vi "LabVIEW Code.vi"() -> ()   [LabVIEW 2017]
uses:
  <vilib>/AWS Toolkit/Core/HTTP Request/AWS Credentials.ctl
  <vilib>/AWS Toolkit/Core/HTTP Request/Region.ctl
  <vilib>/Utility/error.llb/DialogType.ctl
  <vilib>/AWS Toolkit/JSON Parsing/JSON Type.ctl
  <vilib>/DAQmx/read.llb/DAQmx Read (Analog 1D Wfm NChan NSamp).vi
  <extravilib>/ChannelInstances/Tag-bool/Read With Abort.vi
  <extravilib>/ChannelInstances/Tag-bool/Write With Abort.vi
  <extravilib>/ChannelInstances/Tag-bool/Instantiate.vi
  <vilib>/VirtualBench/_PS Configure Voltage Output2.vi
  <vilib>/VirtualBench/_PS Configure Voltage Output1.vi
  <vilib>/VirtualBench/_DMM Configure Measurement6.vi
  <vilib>/VirtualBench/_FGEN Configure Standard Waveform30.vi
  <vilib>/Waveform/WDTFileIO.llb/Export Waveforms To Spreadsheet File (1D).vi
  <vilib>/DAQmx/create/channels.llb/DAQmx Create Channel (AI-Voltage-Basic).vi
  <vilib>/DAQmx/configure/timing.llb/DAQmx Timing (Sample Clock).vi
  <vilib>/DAQmx/miscellaneous.llb/DAQmx Fill In Error Info.vi
  <extravilib>/ChannelInstances/Tag-bool/EndpointRead.vi
  <extravilib>/ChannelInstances/Tag-bool/Endpoint.vi
  <vilib>/AWS Toolkit/IoT/IoT Session/IoT Session.lvclass
  <vilib>/AWS Toolkit/Core/HTTP Request/HTTP Request.lvclass
  <vilib>/AWS Toolkit/IoT/Thing Shadow/Thing Shadow.lvclass
  <vilib>/AWS Toolkit/JSON Parsing/NI_JSON Parsing.lvlib
  <vilib>/VirtualBench/VirtualBench.lvlib
  <extravilib>/ChannelInstances/Tag-bool.lvlib
panel:
  in  "Physical Channel":tag="Dev1/ai0"
  out "usbAcquire":string
  out "Reset":string
  out "msoAcquire":string
  out "VB Name":string="False"
  out "FGen Waveform":string="False"
  out "FGen Waveform":i32
  out "DMM Measurement":dbl caption="Measurement"
  out "DIOUpdateValue":string
  out "DIOPins":tag
  out "pin 7":string
  out "pin 6":string
  out "pin 5":string
  out "pin 4":string
  out "pin 3":string
  out "pin 2":string
  out "pin 1":string
  out "pin 0":string
  out "stopProgramme":string
  out "Alexa Stop":bool=TRUE
  out "DMM Range":dbl caption="Range"
  out "Needs Updating":bool=TRUE
  out "Device Name":tag="VB8012-308BD6C"
  out "Current Update Value":dbl
  out "Update":i32
  out "Voltage Update Value":dbl
  out "Voltage Channel":tag="ps/+6V"
  in  "Auto Range":bool=TRUE
  out "DMM Function String":string
  in  "DMM Function":i32
  out "Current C1":dbl
  out "Current C3":dbl
  out "Current C2":dbl
  out "Voltage C3":dbl
  out "Voltage C2":dbl
  out "Voltage C1":dbl
  out "output string":string
  in  "stop":bool
  out "Raw JSON":string
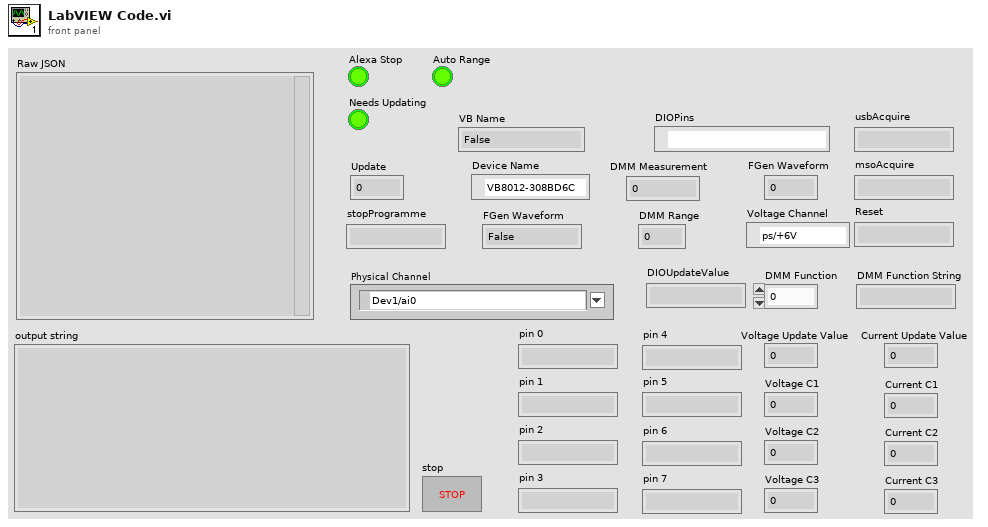
[diagram p1: front panel]
types:
  T1 = typedef "NI_AWS_Core.lvlib/HTTP Request.lvclass/Region.ctl" = enum16{"us-east-1", "us-east-2", "us-west-1", "us-west-2", "ap-northeast-1", "ap-northeast-2", "ap-southeast-1", "ap-southeast-2", "ca-central-1", "eu-central-1", "eu-west-1", "eu-west-2", "sa-east-1"}
  T2 = typedef "NI_AWS_Core.lvlib/HTTP Request.lvclass/AWS Credentials.ctl" = cluster{"Access Key":string, "Secret Key":string}
  T3 = typedef "NI_JSON Parsing.lvlib/JSON Type.ctl" = enum16{"String", "Numeric", "Boolean"}
  T4 = typedef "NI_JSON Parsing.lvlib/Name-Value with Type.ctl" = cluster{"Name Value Pair":T5, "JSON Type":T3}
  T5 = typedef "NI_JSON Parsing.lvlib/Name Value Pair.ctl" = cluster{"name":string, "value":string}
  T6 = cluster{cluster{string, "NumText.Text":string}, "JSON Type":T3}
  T7 = cluster{cluster{string, "NumText.Text":string}, "JSON Type":T3}[]
  T8 = cluster{cluster{string, "DMM Function String":string}, "JSON Type":T3}
  T9 = cluster{cluster{string, "DMM Function String":string}, "JSON Type":T3}[]
  T10 = cluster{cluster{string, string}, "JSON Type":T3}[]
  T11 = cluster{cluster{string, "pin 0":string}, "JSON Type":T3}
  T12 = cluster{cluster{string, "pin 0":string}, "JSON Type":T3}[]
  T13 = cluster{cluster{string, "pin 1":string}, "JSON Type":T3}
  T14 = cluster{cluster{string, "pin 1":string}, "JSON Type":T3}[]
  T15 = cluster{cluster{string, "pin 2":string}, "JSON Type":T3}
  T16 = cluster{cluster{string, "pin 2":string}, "JSON Type":T3}[]
  T17 = cluster{cluster{string, "pin 3":string}, "JSON Type":T3}
  T18 = cluster{cluster{string, "pin 3":string}, "JSON Type":T3}[]
  T19 = cluster{cluster{string, "pin 4":string}, "JSON Type":T3}
  T20 = cluster{cluster{string, "pin 4":string}, "JSON Type":T3}[]
  T21 = cluster{cluster{string, "pin 5":string}, "JSON Type":T3}
  T22 = cluster{cluster{string, "pin 5":string}, "JSON Type":T3}[]
  T23 = cluster{cluster{string, "pin 6":string}, "JSON Type":T3}
  T24 = cluster{cluster{string, "pin 6":string}, "JSON Type":T3}[]
  T25 = cluster{cluster{string, "pin 7":string}, "JSON Type":T3}
  T26 = cluster{cluster{string, "pin 7":string}, "JSON Type":T3}[]
  T27 = cluster{cluster{string, "msoAcquire":string}, "JSON Type":T3}
  T28 = cluster{cluster{string, "msoAcquire":string}, "JSON Type":T3}[]
  T29 = cluster{cluster{string, "usbAcquire":string}, "JSON Type":T3}
  T30 = cluster{cluster{string, "usbAcquire":string}, "JSON Type":T3}[]
  T31 = cluster{cluster{string, "Reset":string}, "JSON Type":T3}
  T32 = cluster{cluster{string, "Reset":string}, "JSON Type":T3}[]
  T33 = cluster{"output string":string, "output string":string}
  T34 = cluster{cluster{"output string":string, "output string":string}, "JSON Type":T3}
  T35 = cluster{cluster{"output string":string, "output string":string}, "JSON Type":T3}[]
  T36 = typedef "Tag-bool.lvlib/))Channel.ctl" = refnum<queue>
  T37 = typedef "DialogType.ctl" = u16
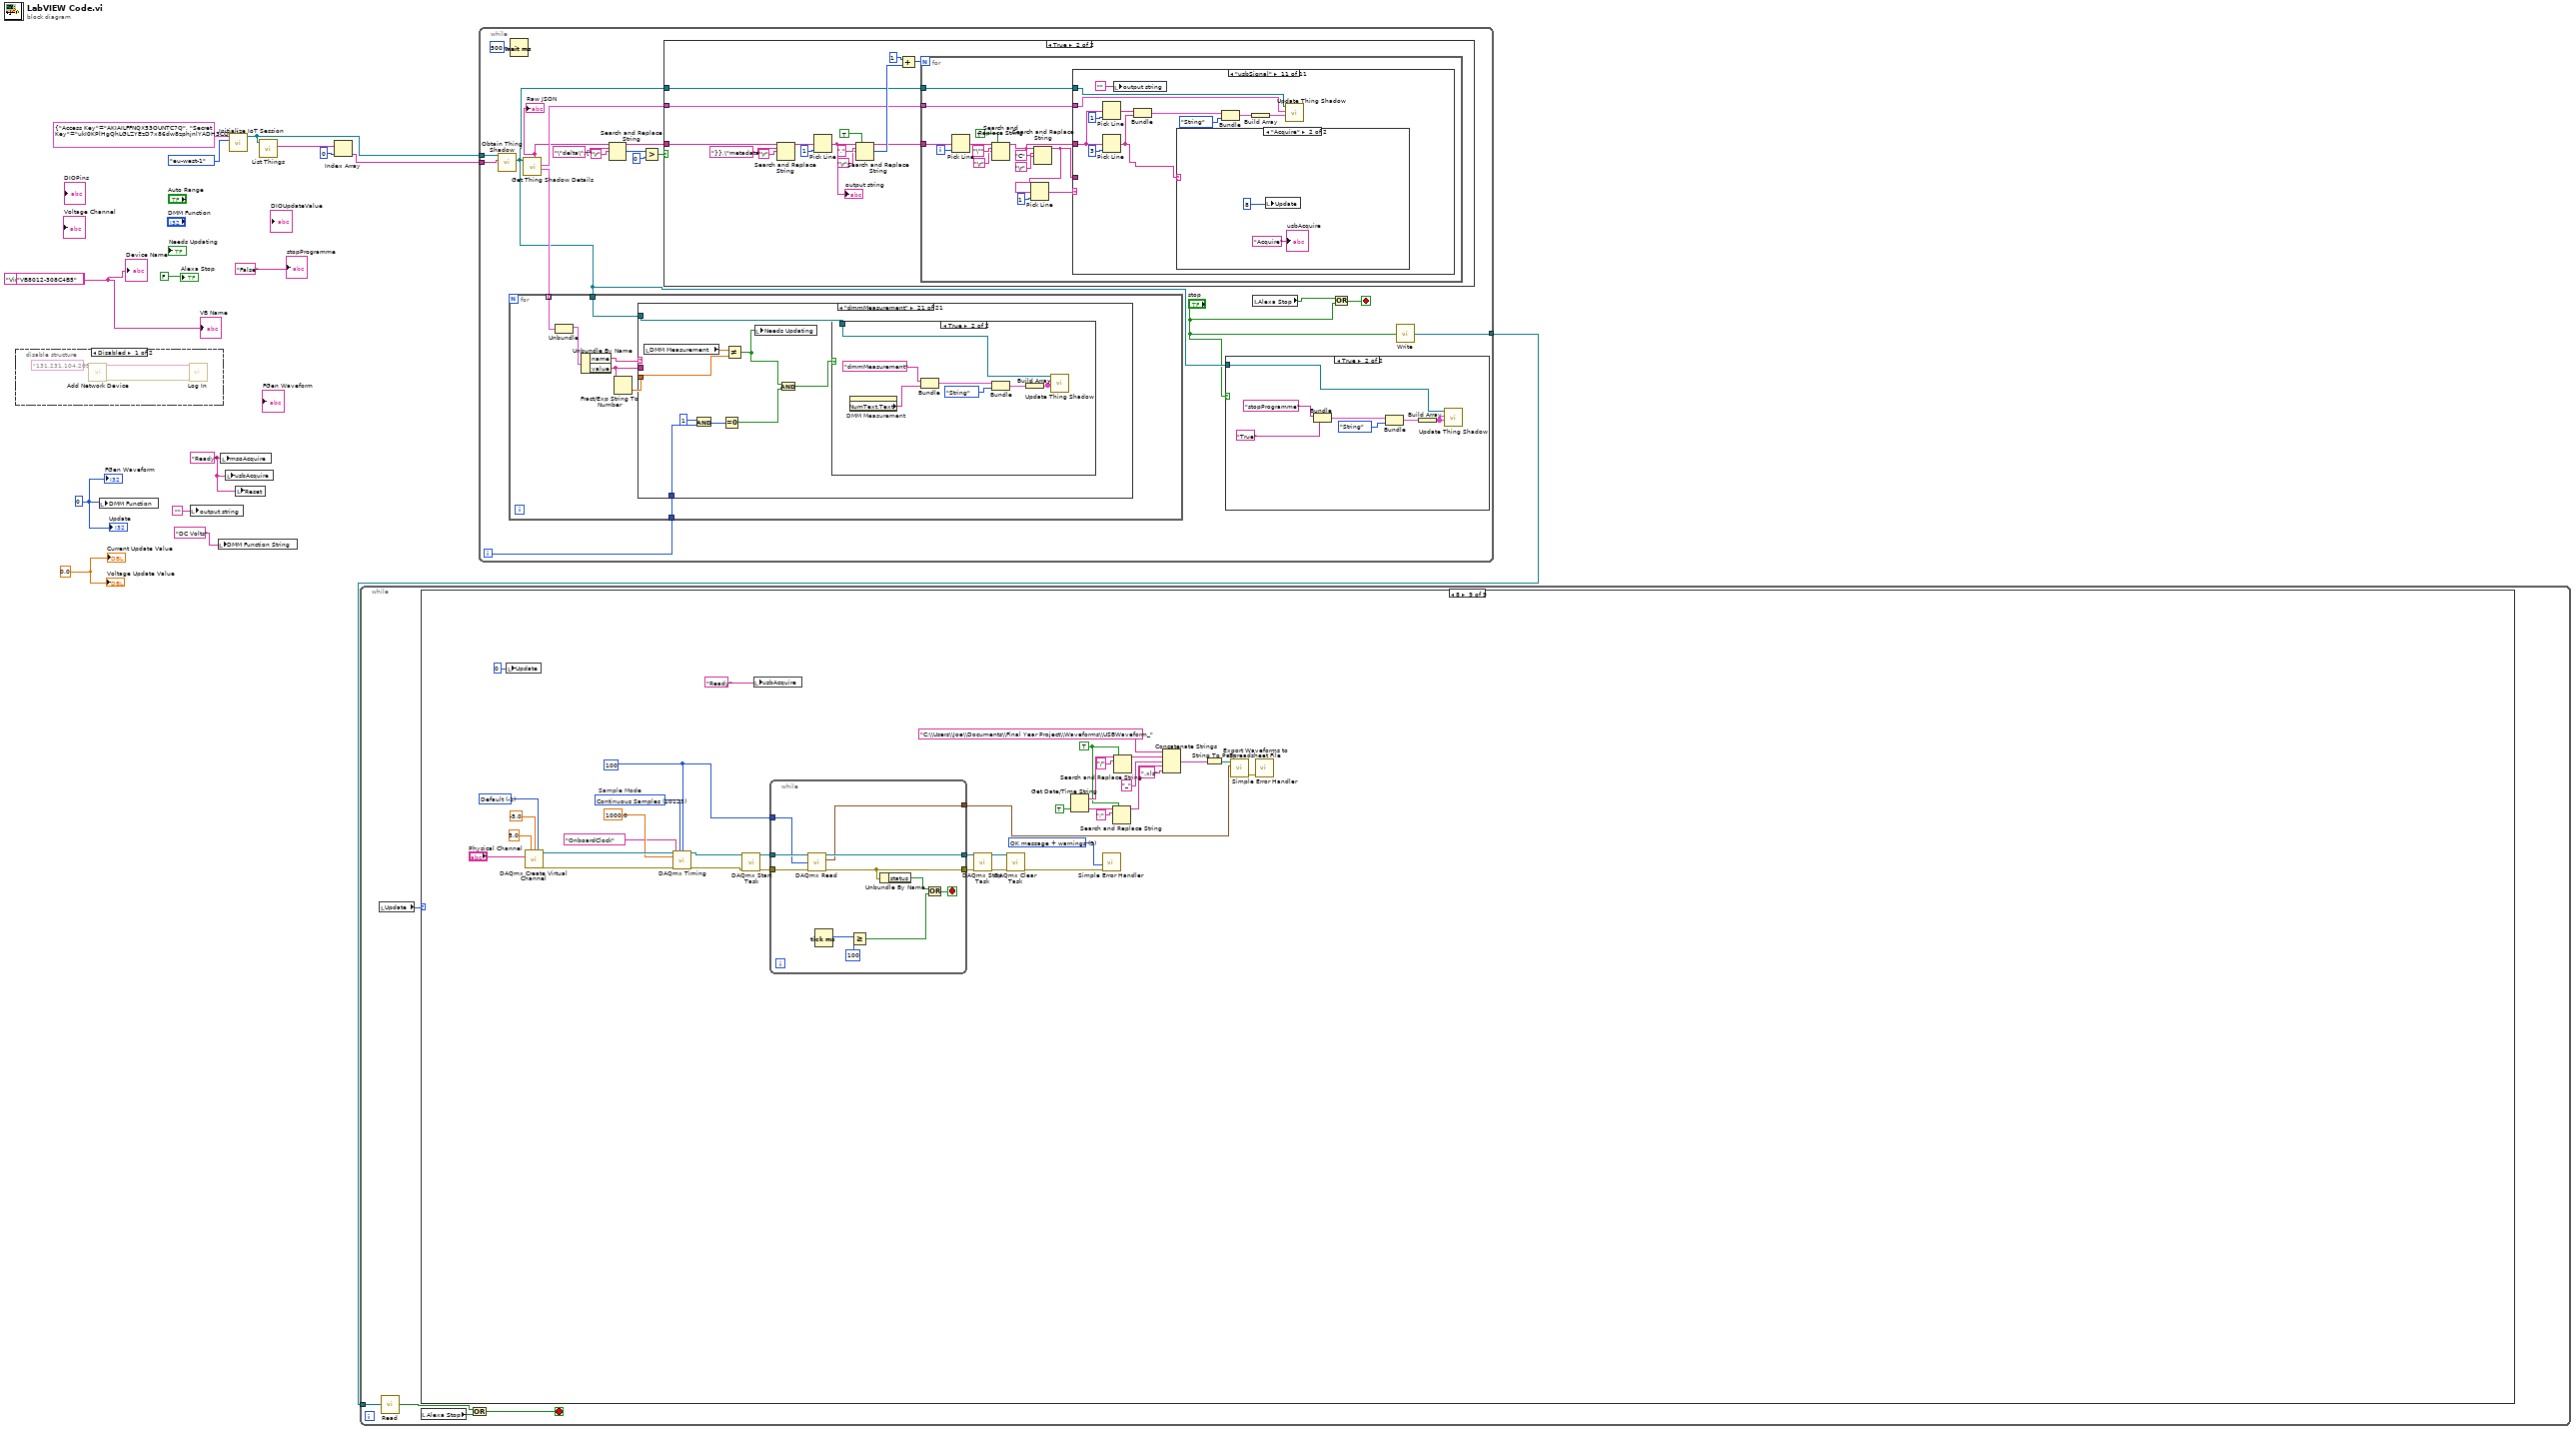
[diagram p0: block diagram]
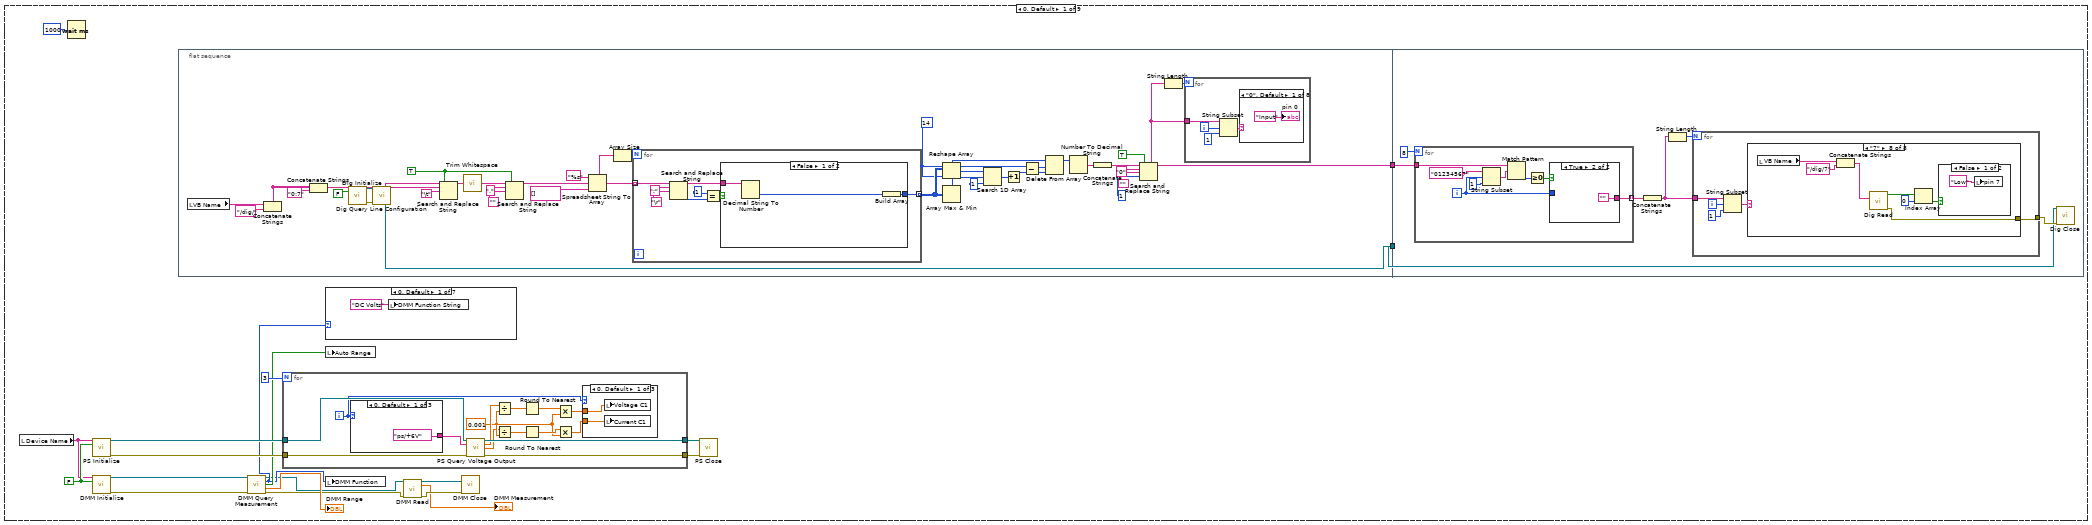
[diagram p3: hidden frame]
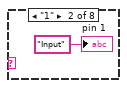
[diagram p4: hidden frame]
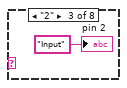
[diagram p5: hidden frame]
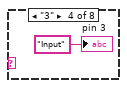
[diagram p6: hidden frame]
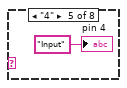
[diagram p7: hidden frame]
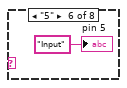
[diagram p8: hidden frame]
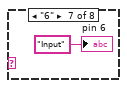
[diagram p9: hidden frame]
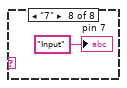
[diagram p10: hidden frame]
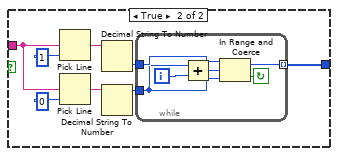
[diagram p11: hidden frame]
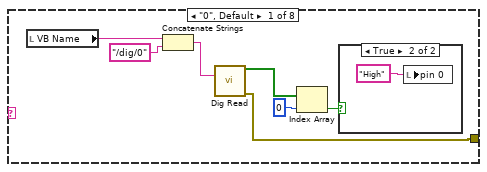
[diagram p12: hidden frame]
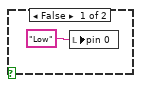
[diagram p13: hidden frame]
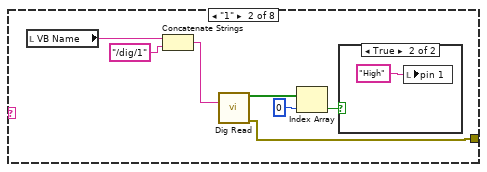
[diagram p14: hidden frame]
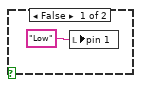
[diagram p15: hidden frame]
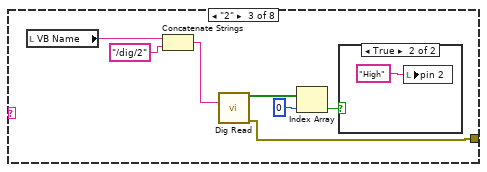
[diagram p16: hidden frame]
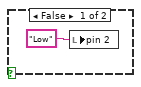
[diagram p17: hidden frame]
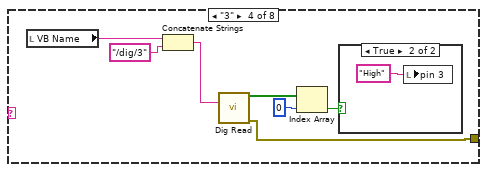
[diagram p18: hidden frame]
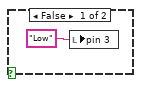
[diagram p19: hidden frame]
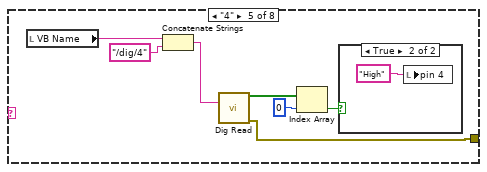
[diagram p20: hidden frame]
diagram:
  w1 = "Ready"
  w2 = tag "VirtualBench-Tank-1" ("Device Name")
  (unwired) tag "VB8012-308C4B5" ("Device Name")
  w8 = 0
  w7 = 0.0
  n1 = disable-structure shown="Disabled" {
    frame Disabled {
      n2 = call <vilib>:"Add Network Device.vi"("IP Or Hostname"="131.231.104.203") -> ("Device"=w18:tag, "Error Out"=w16:errorcluster)  [unwired: 13 in]
      n3 = call <vilib>:"Log In.vi"("Device"=w18, "Error In"=w16) -> ()  [unwired: 13 in, 1 out]
    }
    frame Enabled {
    }
  }
  n4 = local write "DMM Function"(w8) -> ()
  n5 = local write "output string"("") -> ()
  n6 = local write "DMM Function String"("DC Volts") -> ()
  n7 = local write "msoAcquire"(w1) -> ()
  n8 = local write "usbAcquire"(w1) -> ()
  n9 = call <vilib>:"Initialize IoT Session.vi"("Region"=Region."eu-west-1", "AWS Credentials"=T2 {"Access Key"="AKIAILFFNQX53OUNTC7Q", "Secret Key"="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"}) -> ("IoT Session"=w10:refnum<class "IoT Session.lvclass">)  [unwired: 8 in, 1 out]
  n10 = local write "Reset"(w1) -> ()
  n11 = call <vilib>:"List Things.vi"("IoT Session in"=w10) -> ("Things"=w13:string[])  [unwired: 8 in, 2 out]
  n12 = Index Array(array=w13, index=0) -> (element=w11:string)
  n13 = while {
    tunnel: w10 -> [w36]
    tunnel: w11 -> [w35]
    tunnel: [w20] -> w3
    i -> [w19]
    stop <- w24 stop-if-true
    n14 = call <vilib>:"Obtain Thing Shadow.vi"("Thing Name"=w35, "IoT Session in"=w36) -> ("Shadow Thing"=w22:refnum<class "Thing Shadow.lvclass">)  [unwired: 7 in, 2 out]
    n15 = Wait (ms)(milliseconds to wait=u32 500) -> ()  [unwired: 1 out]
    n16 = call <vilib>:"Get Thing Shadow Details.vi"("Thing Shadow in"=w22) -> ("Reported State"=w26:T4[], "Desired State"=w27:T4[], "Raw JSON"=w25:string)  [unwired: 5 in, 3 out]
    "Raw JSON" <- w25
    n17 = for {
      tunnel: w26 -> [w50] mode=indexing
      tunnel: w22 -> [w46]
      tunnel: w19 -> [w44]
      n18 = Unbundle(w50) -> ("Name Value Pair"=w49:T5)  [unwired: 1 out]
      n19 = Unbundle By Name(w49) -> ("name"=w48:string, "value"=w45:string)
      n20 = Fract/Exp String To Number(string=w45) -> (number=w47:dbl)  [unwired: 3 in, 1 out]
      n21 = case shown="\"dmmMeasurement\"" w48 {
        tunnel: w47 -> [_ w53 w64 w75 w86 w97 w108 _ _ _ _ _ _ _ _ _ _ _ _ _ w315]
        tunnel: w46 -> [_ w51 w62 w73 w84 w95 w106 w118 w133 w148 w163 w178 w193 w208 w223 w238 w253 w268 w283 w298 w314]
        tunnel: w45 -> [_ _ _ _ _ _ _ w117 w132 w147 w162 w177 w192 w207 w222 w237 w252 w267 w282 w297 _]
        tunnel: w44 -> [_ _ _ _ _ _ _ _ _ _ _ _ _ _ _ _ _ _ _ _ w313]
        frame "j", Default {
        }
        frame "voltageC1" {
          n22 = local read "Voltage C1"() -> (w54:dbl)
          n23 = Not Equal?(x=w54, y=w53) -> (x != y?=w52:bool)
          n24 = local write "Needs Updating"(w52) -> ()
          n25 = case shown="True" w52 {
            tunnel: w51 -> [_ w57]
            frame False {
            }
            frame True {
              n26 = property on="Voltage C1" class="DigNum (strict)"() -> ("NumText.Text"=w56:string)  [unwired: 2 in, 2 out]
              n27 = Bundle("voltageC1", "NumText.Text"=w56) -> (w59:cluster{string, "NumText.Text":string})  [unwired: 1 in]
              n28 = Bundle(w59, "JSON Type"=JSON_Type."String") -> (w58:T6)  [unwired: 1 in]
              n29 = Build Array(w58) -> (w61:T7)
              n30 = call <vilib>:"Update Thing Shadow.vi"("Reported State"=w61, "Desired State"=w61, "Thing Shadow in"=w57) -> ()  [unwired: 7 in, 2 out]
            }
          }
        }
        frame "voltageC2" {
          n31 = local read "Voltage C2"() -> (w65:dbl)
          n32 = Not Equal?(x=w65, y=w64) -> (x != y?=w63:bool)
          n33 = local write "Needs Updating"(w63) -> ()
          n34 = case shown="False" w63 {
            tunnel: w62 -> [_ w68]
            frame False {
            }
            frame True {
              n35 = property on="Voltage C2" class="DigNum (strict)"() -> ("NumText.Text"=w67:string)  [unwired: 2 in, 2 out]
              n36 = Bundle("voltageC2", "NumText.Text"=w67) -> (w70:cluster{string, "NumText.Text":string})  [unwired: 1 in]
              n37 = Bundle(w70, "JSON Type"=JSON_Type."String") -> (w69:T6)  [unwired: 1 in]
              n38 = Build Array(w69) -> (w72:T7)
              n39 = call <vilib>:"Update Thing Shadow.vi"("Reported State"=w72, "Desired State"=w72, "Thing Shadow in"=w68) -> ()  [unwired: 7 in, 2 out]
            }
          }
        }
        frame "voltageC3" {
          n40 = local read "Voltage C3"() -> (w76:dbl)
          n41 = Not Equal?(x=w76, y=w75) -> (x != y?=w74:bool)
          n42 = local write "Needs Updating"(w74) -> ()
          n43 = case shown="True" w74 {
            tunnel: w73 -> [_ w79]
            frame False {
            }
            frame True {
              n44 = property on="Voltage C3" class="DigNum (strict)"() -> ("NumText.Text"=w78:string)  [unwired: 2 in, 2 out]
              n45 = Bundle("voltageC3", "NumText.Text"=w78) -> (w81:cluster{string, "NumText.Text":string})  [unwired: 1 in]
              n46 = Bundle(w81, "JSON Type"=JSON_Type."String") -> (w80:T6)  [unwired: 1 in]
              n47 = Build Array(w80) -> (w83:T7)
              n48 = call <vilib>:"Update Thing Shadow.vi"("Reported State"=w83, "Desired State"=w83, "Thing Shadow in"=w79) -> ()  [unwired: 7 in, 2 out]
            }
          }
        }
        frame "currentC1" {
          n49 = local read "Current C1"() -> (w87:dbl)
          n50 = Not Equal?(x=w87, y=w86) -> (x != y?=w85:bool)
          n51 = local write "Needs Updating"(w85) -> ()
          n52 = case shown="True" w85 {
            tunnel: w84 -> [_ w90]
            frame False {
            }
            frame True {
              n53 = property on="Current C1" class="DigNum (strict)"() -> ("NumText.Text"=w89:string)  [unwired: 2 in, 2 out]
              n54 = Bundle("currentC1", "NumText.Text"=w89) -> (w92:cluster{string, "NumText.Text":string})  [unwired: 1 in]
              n55 = Bundle(w92, "JSON Type"=JSON_Type."String") -> (w91:T6)  [unwired: 1 in]
              n56 = Build Array(w91) -> (w94:T7)
              n57 = call <vilib>:"Update Thing Shadow.vi"("Reported State"=w94, "Desired State"=w94, "Thing Shadow in"=w90) -> ()  [unwired: 7 in, 2 out]
            }
          }
        }
        frame "currentC2" {
          n58 = local read "Current C2"() -> (w98:dbl)
          n59 = Not Equal?(x=w98, y=w97) -> (x != y?=w96:bool)
          n60 = local write "Needs Updating"(w96) -> ()
          n61 = case shown="True" w96 {
            tunnel: w95 -> [_ w101]
            frame False {
            }
            frame True {
              n62 = property on="Current C2" class="DigNum (strict)"() -> ("NumText.Text"=w100:string)  [unwired: 2 in, 2 out]
              n63 = Bundle("currentC2", "NumText.Text"=w100) -> (w103:cluster{string, "NumText.Text":string})  [unwired: 1 in]
              n64 = Bundle(w103, "JSON Type"=JSON_Type."String") -> (w102:T6)  [unwired: 1 in]
              n65 = Build Array(w102) -> (w105:T7)
              n66 = call <vilib>:"Update Thing Shadow.vi"("Reported State"=w105, "Desired State"=w105, "Thing Shadow in"=w101) -> ()  [unwired: 7 in, 2 out]
            }
          }
        }
        frame "currentC3" {
          n67 = local read "Current C3"() -> (w109:dbl)
          n68 = Not Equal?(x=w109, y=w108) -> (x != y?=w107:bool)
          n69 = local write "Needs Updating"(w107) -> ()
          n70 = case shown="True" w107 {
            tunnel: w106 -> [_ w110]
            frame False {
            }
            frame True {
              n71 = property on="Current C3" class="DigNum (strict)"() -> ("NumText.Text"=w112:string)  [unwired: 2 in, 2 out]
              n72 = Bundle("currentC3", "NumText.Text"=w112) -> (w114:cluster{string, "NumText.Text":string})  [unwired: 1 in]
              n73 = Bundle(w114, "JSON Type"=JSON_Type."String") -> (w113:T6)  [unwired: 1 in]
              n74 = Build Array(w113) -> (w116:T7)
              n75 = call <vilib>:"Update Thing Shadow.vi"("Reported State"=w116, "Desired State"=w116, "Thing Shadow in"=w110) -> ()  [unwired: 7 in, 2 out]
            }
          }
        }
        frame "dmmFunction" {
          n76 = local read "DMM Function String"() -> (w120:string)
          n77 = Not Equal?(x=w120, y=w117) -> (x != y?=w119:bool)
          n78 = local write "Needs Updating"(w119) -> ()
          n79 = case shown="True" w119 {
            tunnel: w118 -> [_ w123]
            frame False {
            }
            frame True {
              n80 = local read "DMM Function String"() -> (w122:string)
              n81 = Bundle("dmmFunction", "DMM Function String"=w122) -> (w126:cluster{string, "DMM Function String":string})  [unwired: 1 in]
              n82 = Bundle(w126, "JSON Type"=JSON_Type."String") -> (w125:T8)  [unwired: 1 in]
              n83 = Build Array(w125) -> (w121:T9)
              n84 = call <vilib>:"Update Thing Shadow.vi"("Reported State"=w121, "Desired State"=w121, "Thing Shadow in"=w123) -> ()  [unwired: 7 in, 2 out]
            }
          }
        }
        frame "stopProgramme" {
          n85 = local read "stopProgramme"() -> (w134:string)
          n86 = local read "Alexa Stop"() -> (w129:bool)
          n87 = Not Equal?(x=w134, y=w132) -> (x != y?=w131:bool)
          n88 = Not(x=w129) -> (.not. x?=w128:bool)
          n89 = local write "Needs Updating"(w131) -> ()
          n90 = And(x=w131, y=w128) -> (x .and. y?=w130:bool)
          n91 = case shown="True" w130 {
            tunnel: w133 -> [_ w138]
            frame False {
            }
            frame True {
              n92 = local write "output string"("") -> ()
              n93 = Bundle("stopProgramme", "False") -> (w141:cluster{string, string})  [unwired: 1 in]
              n94 = Bundle(w141, "JSON Type"=JSON_Type."String") -> (w140:cluster{cluster{string, string}, "JSON Type":T3})  [unwired: 1 in]
              n95 = Build Array(w140) -> (w137:T10)
              n96 = call <vilib>:"Update Thing Shadow.vi"("Reported State"=w137, "Desired State"=w137, "Thing Shadow in"=w138) -> ()  [unwired: 7 in, 2 out]
            }
          }
        }
        frame "pinC0" {
          n97 = local read "Alexa Stop"() -> (w144:bool)
          n98 = local read "pin 0"() -> (w149:string)
          n99 = Not Equal?(x=w149, y=w147) -> (x != y?=w146:bool)
          n100 = Not(x=w144) -> (.not. x?=w143:bool)
          n101 = local write "Needs Updating"(w146) -> ()
          n102 = And(x=w146, y=w143) -> (x .and. y?=w145:bool)
          n103 = case shown="True" w145 {
            tunnel: w148 -> [_ w157]
            frame False {
            }
            frame True {
              n104 = local read "pin 0"() -> (w150:string)
              n105 = local write "output string"("") -> ()
              n106 = Bundle("pinC0", "pin 0"=w150) -> (w155:cluster{string, "pin 0":string})  [unwired: 1 in]
              n107 = Bundle(w155, "JSON Type"=JSON_Type."String") -> (w154:T11)  [unwired: 1 in]
              n108 = Build Array(w154) -> (w152:T12)
              n109 = call <vilib>:"Update Thing Shadow.vi"("Reported State"=w152, "Desired State"=w152, "Thing Shadow in"=w157) -> ()  [unwired: 7 in, 2 out]
            }
          }
        }
        frame "pinC1" {
          n110 = local read "Alexa Stop"() -> (w159:bool)
          n111 = local read "pin 1"() -> (w164:string)
          n112 = Not Equal?(x=w164, y=w162) -> (x != y?=w161:bool)
          n113 = Not(x=w159) -> (.not. x?=w158:bool)
          n114 = local write "Needs Updating"(w161) -> ()
          n115 = And(x=w161, y=w158) -> (x .and. y?=w160:bool)
          n116 = case shown="True" w160 {
            tunnel: w163 -> [_ w168]
            frame False {
            }
            frame True {
              n117 = local read "pin 1"() -> (w165:string)
              n118 = local write "output string"("") -> ()
              n119 = Bundle("pinC1", "pin 1"=w165) -> (w171:cluster{string, "pin 1":string})  [unwired: 1 in]
              n120 = Bundle(w171, "JSON Type"=JSON_Type."String") -> (w170:T13)  [unwired: 1 in]
              n121 = Build Array(w170) -> (w167:T14)
              n122 = call <vilib>:"Update Thing Shadow.vi"("Reported State"=w167, "Desired State"=w167, "Thing Shadow in"=w168) -> ()  [unwired: 7 in, 2 out]
            }
          }
        }
        frame "pinC2" {
          n123 = local read "Alexa Stop"() -> (w174:bool)
          n124 = local read "pin 2"() -> (w179:string)
          n125 = Not Equal?(x=w179, y=w177) -> (x != y?=w176:bool)
          n126 = Not(x=w174) -> (.not. x?=w173:bool)
          n127 = local write "Needs Updating"(w176) -> ()
          n128 = And(x=w176, y=w173) -> (x .and. y?=w175:bool)
          n129 = case shown="True" w175 {
            tunnel: w178 -> [_ w183]
            frame False {
            }
            frame True {
              n130 = local read "pin 2"() -> (w180:string)
              n131 = local write "output string"("") -> ()
              n132 = Bundle("pinC2", "pin 2"=w180) -> (w186:cluster{string, "pin 2":string})  [unwired: 1 in]
              n133 = Bundle(w186, "JSON Type"=JSON_Type."String") -> (w185:T15)  [unwired: 1 in]
              n134 = Build Array(w185) -> (w182:T16)
              n135 = call <vilib>:"Update Thing Shadow.vi"("Reported State"=w182, "Desired State"=w182, "Thing Shadow in"=w183) -> ()  [unwired: 7 in, 2 out]
            }
          }
        }
        frame "pinC3" {
          n136 = local read "Alexa Stop"() -> (w189:bool)
          n137 = local read "pin 3"() -> (w194:string)
          n138 = Not Equal?(x=w194, y=w192) -> (x != y?=w191:bool)
          n139 = Not(x=w189) -> (.not. x?=w188:bool)
          n140 = local write "Needs Updating"(w191) -> ()
          n141 = And(x=w191, y=w188) -> (x .and. y?=w190:bool)
          n142 = case shown="True" w190 {
            tunnel: w193 -> [_ w198]
            frame False {
            }
            frame True {
              n143 = local read "pin 3"() -> (w195:string)
              n144 = local write "output string"("") -> ()
              n145 = Bundle("pinC3", "pin 3"=w195) -> (w201:cluster{string, "pin 3":string})  [unwired: 1 in]
              n146 = Bundle(w201, "JSON Type"=JSON_Type."String") -> (w200:T17)  [unwired: 1 in]
              n147 = Build Array(w200) -> (w197:T18)
              n148 = call <vilib>:"Update Thing Shadow.vi"("Reported State"=w197, "Desired State"=w197, "Thing Shadow in"=w198) -> ()  [unwired: 7 in, 2 out]
            }
          }
        }
        frame "pinC4" {
          n149 = local read "Alexa Stop"() -> (w204:bool)
          n150 = local read "pin 4"() -> (w209:string)
          n151 = Not Equal?(x=w209, y=w207) -> (x != y?=w206:bool)
          n152 = Not(x=w204) -> (.not. x?=w203:bool)
          n153 = local write "Needs Updating"(w206) -> ()
          n154 = And(x=w206, y=w203) -> (x .and. y?=w205:bool)
          n155 = case shown="True" w205 {
            tunnel: w208 -> [_ w213]
            frame False {
            }
            frame True {
              n156 = local read "pin 4"() -> (w210:string)
              n157 = local write "output string"("") -> ()
              n158 = Bundle("pinC4", "pin 4"=w210) -> (w216:cluster{string, "pin 4":string})  [unwired: 1 in]
              n159 = Bundle(w216, "JSON Type"=JSON_Type."String") -> (w215:T19)  [unwired: 1 in]
              n160 = Build Array(w215) -> (w212:T20)
              n161 = call <vilib>:"Update Thing Shadow.vi"("Reported State"=w212, "Desired State"=w212, "Thing Shadow in"=w213) -> ()  [unwired: 7 in, 2 out]
            }
          }
        }
        frame "pinC5" {
          n162 = local read "Alexa Stop"() -> (w219:bool)
          n163 = local read "pin 5"() -> (w224:string)
          n164 = Not Equal?(x=w224, y=w222) -> (x != y?=w221:bool)
          n165 = Not(x=w219) -> (.not. x?=w218:bool)
          n166 = local write "Needs Updating"(w221) -> ()
          n167 = And(x=w221, y=w218) -> (x .and. y?=w220:bool)
          n168 = case shown="True" w220 {
            tunnel: w223 -> [_ w228]
            frame False {
            }
            frame True {
              n169 = local read "pin 5"() -> (w225:string)
              n170 = local write "output string"("") -> ()
              n171 = Bundle("pinC5", "pin 5"=w225) -> (w231:cluster{string, "pin 5":string})  [unwired: 1 in]
              n172 = Bundle(w231, "JSON Type"=JSON_Type."String") -> (w230:T21)  [unwired: 1 in]
              n173 = Build Array(w230) -> (w227:T22)
              n174 = call <vilib>:"Update Thing Shadow.vi"("Reported State"=w227, "Desired State"=w227, "Thing Shadow in"=w228) -> ()  [unwired: 7 in, 2 out]
            }
          }
        }
        frame "pinC6" {
          n175 = local read "Alexa Stop"() -> (w234:bool)
          n176 = local read "pin 6"() -> (w239:string)
          n177 = Not Equal?(x=w239, y=w237) -> (x != y?=w236:bool)
          n178 = Not(x=w234) -> (.not. x?=w233:bool)
          n179 = local write "Needs Updating"(w236) -> ()
          n180 = And(x=w236, y=w233) -> (x .and. y?=w235:bool)
          n181 = case shown="True" w235 {
            tunnel: w238 -> [_ w243]
            frame False {
            }
            frame True {
              n182 = local read "pin 6"() -> (w240:string)
              n183 = local write "output string"("") -> ()
              n184 = Bundle("pinC6", "pin 6"=w240) -> (w246:cluster{string, "pin 6":string})  [unwired: 1 in]
              n185 = Bundle(w246, "JSON Type"=JSON_Type."String") -> (w245:T23)  [unwired: 1 in]
              n186 = Build Array(w245) -> (w242:T24)
              n187 = call <vilib>:"Update Thing Shadow.vi"("Reported State"=w242, "Desired State"=w242, "Thing Shadow in"=w243) -> ()  [unwired: 7 in, 2 out]
            }
          }
        }
        frame "pinC7" {
          n188 = local read "Alexa Stop"() -> (w249:bool)
          n189 = local read "pin 7"() -> (w254:string)
          n190 = Not Equal?(x=w254, y=w252) -> (x != y?=w251:bool)
          n191 = Not(x=w249) -> (.not. x?=w248:bool)
          n192 = local write "Needs Updating"(w251) -> ()
          n193 = And(x=w251, y=w248) -> (x .and. y?=w250:bool)
          n194 = case shown="True" w250 {
            tunnel: w253 -> [_ w258]
            frame False {
            }
            frame True {
              n195 = local read "pin 7"() -> (w255:string)
              n196 = local write "output string"("") -> ()
              n197 = Bundle("pinC7", "pin 7"=w255) -> (w261:cluster{string, "pin 7":string})  [unwired: 1 in]
              n198 = Bundle(w261, "JSON Type"=JSON_Type."String") -> (w260:T25)  [unwired: 1 in]
              n199 = Build Array(w260) -> (w257:T26)
              n200 = call <vilib>:"Update Thing Shadow.vi"("Reported State"=w257, "Desired State"=w257, "Thing Shadow in"=w258) -> ()  [unwired: 7 in, 2 out]
            }
          }
        }
        frame "msoSignal" {
          n201 = local read "msoAcquire"() -> (w269:string)
          n202 = local read "Alexa Stop"() -> (w264:bool)
          n203 = Not Equal?(x=w269, y=w267) -> (x != y?=w266:bool)
          n204 = Not(x=w264) -> (.not. x?=w263:bool)
          n205 = local write "Needs Updating"(w266) -> ()
          n206 = And(x=w266, y=w263) -> (x .and. y?=w265:bool)
          n207 = case shown="True" w265 {
            tunnel: w268 -> [_ w273]
            frame False {
            }
            frame True {
              n208 = local read "msoAcquire"() -> (w270:string)
              n209 = local write "output string"("") -> ()
              n210 = Bundle("msoSignal", "msoAcquire"=w270) -> (w276:cluster{string, "msoAcquire":string})  [unwired: 1 in]
              n211 = Bundle(w276, "JSON Type"=JSON_Type."String") -> (w275:T27)  [unwired: 1 in]
              n212 = Build Array(w275) -> (w272:T28)
              n213 = call <vilib>:"Update Thing Shadow.vi"("Reported State"=w272, "Desired State"=w272, "Thing Shadow in"=w273) -> ()  [unwired: 7 in, 2 out]
            }
          }
        }
        frame "usbSignal" {
          n214 = local read "usbAcquire"() -> (w284:string)
          n215 = local read "Alexa Stop"() -> (w279:bool)
          n216 = Not Equal?(x=w284, y=w282) -> (x != y?=w281:bool)
          n217 = Not(x=w279) -> (.not. x?=w278:bool)
          n218 = local write "Needs Updating"(w281) -> ()
          n219 = And(x=w281, y=w278) -> (x .and. y?=w280:bool)
          n220 = case shown="True" w280 {
            tunnel: w283 -> [_ w288]
            frame False {
            }
            frame True {
              n221 = local read "usbAcquire"() -> (w285:string)
              n222 = local write "output string"("") -> ()
              n223 = Bundle("usbSignal", "usbAcquire"=w285) -> (w291:cluster{string, "usbAcquire":string})  [unwired: 1 in]
              n224 = Bundle(w291, "JSON Type"=JSON_Type."String") -> (w290:T29)  [unwired: 1 in]
              n225 = Build Array(w290) -> (w287:T30)
              n226 = call <vilib>:"Update Thing Shadow.vi"("Reported State"=w287, "Desired State"=w287, "Thing Shadow in"=w288) -> ()  [unwired: 7 in, 2 out]
            }
          }
        }
        frame "reset" {
          n227 = local read "Alexa Stop"() -> (w294:bool)
          n228 = local read "Reset"() -> (w299:string)
          n229 = Not Equal?(x=w299, y=w297) -> (x != y?=w296:bool)
          n230 = Not(x=w294) -> (.not. x?=w293:bool)
          n231 = local write "Needs Updating"(w296) -> ()
          n232 = And(x=w296, y=w293) -> (x .and. y?=w295:bool)
          n233 = case shown="True" w295 {
            tunnel: w298 -> [_ w303]
            frame False {
            }
            frame True {
              n234 = local read "Reset"() -> (w300:string)
              n235 = local write "output string"("") -> ()
              n236 = Bundle("reset", "Reset"=w300) -> (w306:cluster{string, "Reset":string})  [unwired: 1 in]
              n237 = Bundle(w306, "JSON Type"=JSON_Type."String") -> (w305:T31)  [unwired: 1 in]
              n238 = Build Array(w305) -> (w302:T32)
              n239 = call <vilib>:"Update Thing Shadow.vi"("Reported State"=w302, "Desired State"=w302, "Thing Shadow in"=w303) -> ()  [unwired: 7 in, 2 out]
            }
          }
        }
        frame "dmmMeasurement" {
          n240 = local read "DMM Measurement"() -> (w316:dbl)
          n241 = And(x=1, y=w313) -> (x .and. y?=w311:i32)
          n242 = Equal To 0?(x=w311) -> (x = 0?=w310:bool)
          n243 = Not Equal?(x=w316, y=w315) -> (x != y?=w309:bool)
          n244 = local write "Needs Updating"(w309) -> ()
          n245 = And(x=w309, y=w310) -> (x .and. y?=w308:bool)
          n246 = case shown="True" w308 {
            tunnel: w314 -> [_ w319]
            frame False {
            }
            frame True {
              n247 = property on="DMM Measurement" class="DigNum (strict)"() -> ("NumText.Text"=w318:string)  [unwired: 2 in, 2 out]
              n248 = Bundle("dmmMeasurement", "NumText.Text"=w318) -> (w321:cluster{string, "NumText.Text":string})  [unwired: 1 in]
              n249 = Bundle(w321, "JSON Type"=JSON_Type."String") -> (w320:T6)  [unwired: 1 in]
              n250 = Build Array(w320) -> (w323:T7)
              n251 = call <vilib>:"Update Thing Shadow.vi"("Reported State"=w323, "Desired State"=w323, "Thing Shadow in"=w319) -> ()  [unwired: 7 in, 2 out]
            }
          }
        }
      }
    }
    n252 = Search and Replace String(input string=w25, search string="\"delta\":{", replace string="\r") -> (result string=w31:string, number of replacements=w30:i32)  [unwired: 5 in, 2 out]
    n253 = Greater?(x=w30, y=0) -> (0:w28:bool)
    n254 = case shown="True" w28 {
      tunnel: w31 -> [_ w336]
      tunnel: w22 -> [_ w325]
      tunnel: w27 -> [_ w324]
      frame False {
      }
      frame True {
        n255 = Search and Replace String(input string=w336, search string="}},\"metadata", replace string="\r") -> (result string=w335:string)  [unwired: 5 in, 3 out]
        n256 = Pick Line(multi-line string=w335, line index=1) -> (output string=w333:string)  [unwired: 1 in]
        "output string" <- w333
        n257 = Search and Replace String(replace all?=TRUE ("replace all? (F)"), input string=w333, search string=",", replace string="\r") -> (result string=w327:string, number of replacements=w330:i32)  [unwired: 4 in, 2 out]
        n258 = Add(x=1, y=w330) -> (x+y=w328:i32)
        n259 = for {
          N: w328 -> [_]
          tunnel: w327 -> [w351]
          tunnel: w325 -> [w346]
          tunnel: w324 -> [w345]
          i -> [w352]
          n260 = Pick Line(multi-line string=w351, line index=w352) -> (output string=w348:string)  [unwired: 1 in]
          n261 = Search and Replace String(replace all?=TRUE ("replace all? (F)"), input string=w348, search string="\"", replace string="\r") -> (result string=w340:string)  [unwired: 4 in, 3 out]
          n262 = Search and Replace String(input string=w340, search string="C", replace string="\r") -> (result string=w339:string)  [unwired: 5 in, 3 out]
          n263 = Pick Line(multi-line string=w339, line index=1) -> (output string=w341:string)  [unwired: 1 in]
          n264 = case shown="\"usbSignal\"" w341 {
            tunnel: w340 -> [_ _ w359 w384 w407 w439 w456 w508 w529 w543 w559]
            tunnel: w346 -> [_ _ w364 w389 w410 w437 w459 w511 w532 w546 w562]
            tunnel: w345 -> [_ _ w363 w388 w409 w436 w458 w510 w531 w545 w561]
            tunnel: w339 -> [_ _ w355 w380 _ _ w452 _ _ _ _]
            frame "False", Default {
            }
            frame "openProgramme" {
              n265 = local write "output string"("") -> ()
            }
            frame "voltage" {
              n266 = Pick Line(multi-line string=w359, line index=1) -> (output string=w357:string)  [unwired: 1 in]
              n267 = Pick Line(multi-line string=w359, line index=3) -> (output string=w360:string)  [unwired: 1 in]
              n268 = local write "output string"("") -> ()
              n269 = Fract/Exp String To Number(string=w360) -> (number=w361:dbl)  [unwired: 3 in, 1 out]
              n270 = Bundle("output string"=w357, "output string"=w360) -> (w367:T33)  [unwired: 1 in]
              n271 = Pick Line(multi-line string=w355, line index=2) -> (output string=w354:string)  [unwired: 1 in]
              n272 = case shown="\"1\"" w354 {
                tunnel: w361 -> [w372 w375 _ w377]
                frame "2" {
                  n273 = local write "Voltage Update Value"(w372) -> ()
                  n274 = local write "Voltage Channel"(tag "ps/+25V" ("Channel")) -> ()
                  n275 = local write "Update"(1) -> ()
                  "Voltage C2" <- w372
                }
                frame "3" {
                  n276 = local write "Voltage Update Value"(w375) -> ()
                  n277 = local write "Voltage Channel"(tag "ps/-25V" ("Channel")) -> ()
                  n278 = local write "Update"(1) -> ()
                  "Voltage C3" <- w375
                }
                frame "j", Default {
                }
                frame "1" {
                  n279 = local write "Voltage Update Value"(w377) -> ()
                  n280 = local write "Voltage Channel"(tag "ps/+6V" ("Channel")) -> ()
                  n281 = local write "Update"(1) -> ()
                  "Voltage C1" <- w377
                }
              }
              n282 = Bundle(w367, "JSON Type"=JSON_Type."String") -> (w368:T34)  [unwired: 1 in]
              n283 = Build Array(w368) -> (w365:T35)
              n284 = call <vilib>:"Update Thing Shadow.vi"("Reported State"=w365, "Desired State"=w363, "Thing Shadow in"=w364) -> ()  [unwired: 7 in, 2 out]
            }
            frame "current" {
              n285 = Pick Line(multi-line string=w384, line index=1) -> (output string=w382:string)  [unwired: 1 in]
              n286 = Pick Line(multi-line string=w384, line index=3) -> (output string=w385:string)  [unwired: 1 in]
              n287 = local write "output string"("") -> ()
              n288 = Fract/Exp String To Number(string=w385) -> (number=w386:dbl)  [unwired: 3 in, 1 out]
              n289 = Bundle("output string"=w382, "output string"=w385) -> (w392:T33)  [unwired: 1 in]
              n290 = Pick Line(multi-line string=w380, line index=2) -> (output string=w379:string)  [unwired: 1 in]
              n291 = case shown="\"2\"" w379 {
                tunnel: w386 -> [w395 w398 _ w403]
                frame "2" {
                  n292 = local write "Current Update Value"(w395) -> ()
                  n293 = local write "Voltage Channel"(tag "ps/+25V" ("Channel")) -> ()
                  n294 = local write "Update"(2) -> ()
                  "Current C2" <- w395
                }
                frame "3" {
                  n295 = local write "Current Update Value"(w398) -> ()
                  n296 = local write "Voltage Channel"(tag "ps/-25V" ("Channel")) -> ()
                  n297 = local write "Update"(2) -> ()
                  "Current C3" <- w398
                }
                frame "j", Default {
                }
                frame "1" {
                  n298 = local write "Current Update Value"(w403) -> ()
                  n299 = local write "Voltage Channel"(tag "ps/+6V" ("Channel")) -> ()
                  n300 = local write "Update"(2) -> ()
                  "Current C1" <- w403
                }
              }
              n301 = Bundle(w392, "JSON Type"=JSON_Type."String") -> (w393:T34)  [unwired: 1 in]
              n302 = Build Array(w393) -> (w390:T35)
              n303 = call <vilib>:"Update Thing Shadow.vi"("Reported State"=w390, "Desired State"=w388, "Thing Shadow in"=w389) -> ()  [unwired: 7 in, 2 out]
            }
            frame "dmmFunction" {
              n304 = Pick Line(multi-line string=w407, line index=1) -> (output string=w405:string)  [unwired: 1 in]
              n305 = Pick Line(multi-line string=w407, line index=3) -> (output string=w404:string)  [unwired: 1 in]
              "DMM Function String" <- w404
              n306 = local write "output string"("") -> ()
              n307 = Bundle("output string"=w405, "output string"=w404) -> (w413:T33)  [unwired: 1 in]
              n308 = case shown="\"Continuity\"" w404 {
                frame "False", Default {
                }
                frame "DC Volts" {
                  n309 = local write "DMM Function"(0) -> ()
                  n310 = local write "Auto Range"(TRUE) -> ()
                  n311 = local write "Update"(3) -> ()
                }
                frame "AC Volts" {
                  n312 = local write "DMM Function"(1) -> ()
                  n313 = local write "Auto Range"(TRUE) -> ()
                  n314 = local write "Update"(3) -> ()
                }
                frame "DC Current" {
                  n315 = local write "DMM Function"(2) -> ()
                  n316 = local write "Auto Range"(TRUE) -> ()
                  n317 = local write "Update"(3) -> ()
                }
                frame "AC Current" {
                  n318 = local write "DMM Function"(3) -> ()
                  n319 = local write "Auto Range"(TRUE) -> ()
                  n320 = local write "Update"(3) -> ()
                }
                frame "Resistance" {
                  n321 = local write "DMM Function"(4) -> ()
                  n322 = local write "Auto Range"(TRUE) -> ()
                  n323 = local write "Update"(3) -> ()
                }
                frame "Diode" {
                  n324 = local write "DMM Function"(5) -> ()
                  n325 = local write "Auto Range"(TRUE) -> ()
                  n326 = local write "Update"(3) -> ()
                }
                frame "Continuity" {
                  n327 = local write "DMM Function"(6) -> ()
                  n328 = local write "Update"(3) -> ()
                }
              }
              n329 = Bundle(w413, "JSON Type"=JSON_Type."String") -> (w414:T34)  [unwired: 1 in]
              n330 = Build Array(w414) -> (w411:T35)
              n331 = call <vilib>:"Update Thing Shadow.vi"("Reported State"=w411, "Desired State"=w409, "Thing Shadow in"=w410) -> ()  [unwired: 7 in, 2 out]
            }
            frame "stopProgramme" {
              n332 = Pick Line(multi-line string=w439, line index=3) -> (output string=w438:string)  [unwired: 1 in]
              n333 = case shown="\"True\"" w438 {
                selector: w438 -> [_ w443]
                tunnel: w437 -> [_ w444]
                tunnel: w436 -> [_ w441]
                frame "False", Default {
                }
                frame "True" {
                  n334 = local write "Alexa Stop"(TRUE) -> ()
                  n335 = Bundle("stopProgramme", w443) -> (w448:cluster{string, string})  [unwired: 1 in]
                  n336 = Bundle(w448, "JSON Type"=JSON_Type."String") -> (w447:cluster{cluster{string, string}, "JSON Type":T3})  [unwired: 1 in]
                  n337 = Build Array(w447) -> (w442:T10)
                  n338 = call <vilib>:"Update Thing Shadow.vi"("Reported State"=w442, "Desired State"=w441, "Thing Shadow in"=w444) -> ()  [unwired: 7 in, 2 out]
                }
              }
            }
            frame "pin" {
              n339 = Pick Line(multi-line string=w456, line index=1) -> (output string=w454:string)  [unwired: 1 in]
              n340 = Pick Line(multi-line string=w456, line index=3) -> (output string=w450:string)  [unwired: 1 in]
              n341 = local write "output string"("") -> ()
              n342 = Bundle("output string"=w454, "output string"=w450) -> (w462:T33)  [unwired: 1 in]
              n343 = Pick Line(multi-line string=w452, line index=2) -> (output string=w451:string)  [unwired: 1 in]
              n344 = case shown="\"1\"" w451 {
                tunnel: w450 -> [_ w468 w473 w478 w483 w488 w493 w498 w503]
                frame "j", Default {
                }
                frame "0" {
                  n345 = local read "Device Name"() -> (w467:tag)
                  n346 = local write "DIOUpdateValue"(w468) -> ()
                  n347 = local write "Update"(4) -> ()
                  n348 = local write "pin 0"(w468) -> ()
                  n349 = Concatenate Strings(w467, "/dig/0" ("string")) -> (w465:string)
                  n350 = local write "DIOPins"(w465) -> ()
                }
                frame "1" {
                  n351 = local read "Device Name"() -> (w472:tag)
                  n352 = local write "DIOUpdateValue"(w473) -> ()
                  n353 = local write "Update"(4) -> ()
                  n354 = local write "pin 1"(w473) -> ()
                  n355 = Concatenate Strings(w472, "/dig/1" ("string")) -> (w470:string)
                  n356 = local write "DIOPins"(w470) -> ()
                }
                frame "2" {
                  n357 = local read "Device Name"() -> (w477:tag)
                  n358 = local write "DIOUpdateValue"(w478) -> ()
                  n359 = local write "Update"(4) -> ()
                  n360 = local write "pin 2"(w478) -> ()
                  n361 = Concatenate Strings(w477, "/dig/2" ("string")) -> (w475:string)
                  n362 = local write "DIOPins"(w475) -> ()
                }
                frame "3" {
                  n363 = local read "Device Name"() -> (w482:tag)
                  n364 = local write "DIOUpdateValue"(w483) -> ()
                  n365 = local write "Update"(4) -> ()
                  n366 = local write "pin 3"(w483) -> ()
                  n367 = Concatenate Strings(w482, "/dig/3" ("string")) -> (w480:string)
                  n368 = local write "DIOPins"(w480) -> ()
                }
                frame "4" {
                  n369 = local read "Device Name"() -> (w487:tag)
                  n370 = local write "DIOUpdateValue"(w488) -> ()
                  n371 = local write "Update"(4) -> ()
                  n372 = local write "pin 4"(w488) -> ()
                  n373 = Concatenate Strings(w487, "/dig/4" ("string")) -> (w485:string)
                  n374 = local write "DIOPins"(w485) -> ()
                }
                frame "5" {
                  n375 = local read "Device Name"() -> (w492:tag)
                  n376 = local write "DIOUpdateValue"(w493) -> ()
                  n377 = local write "Update"(4) -> ()
                  n378 = local write "pin 5"(w493) -> ()
                  n379 = Concatenate Strings(w492, "/dig/5" ("string")) -> (w490:string)
                  n380 = local write "DIOPins"(w490) -> ()
                }
                frame "6" {
                  n381 = local read "Device Name"() -> (w497:tag)
                  n382 = local write "DIOUpdateValue"(w498) -> ()
                  n383 = local write "Update"(4) -> ()
                  n384 = local write "pin 6"(w498) -> ()
                  n385 = Concatenate Strings(w497, "/dig/6" ("string")) -> (w495:string)
                  n386 = local write "DIOPins"(w495) -> ()
                }
                frame "7" {
                  n387 = local read "Device Name"() -> (w502:tag)
                  n388 = local write "DIOUpdateValue"(w503) -> ()
                  n389 = local write "Update"(4) -> ()
                  n390 = local write "pin 7"(w503) -> ()
                  n391 = Concatenate Strings(w502, "/dig/7" ("string")) -> (w501:string)
                  n392 = local write "DIOPins"(w501) -> ()
                }
              }
              n393 = Bundle(w462, "JSON Type"=JSON_Type."String") -> (w463:T34)  [unwired: 1 in]
              n394 = Build Array(w463) -> (w460:T35)
              n395 = call <vilib>:"Update Thing Shadow.vi"("Reported State"=w460, "Desired State"=w458, "Thing Shadow in"=w459) -> ()  [unwired: 7 in, 2 out]
            }
            frame "fgSignal" {
              n396 = Pick Line(multi-line string=w508, line index=1) -> (output string=w506:string)  [unwired: 1 in]
              n397 = Pick Line(multi-line string=w508, line index=3) -> (output string=w505:string)  [unwired: 1 in]
              n398 = local write "output string"("") -> ()
              n399 = Bundle("output string"=w506, "output string"=w505) -> (w514:T33)  [unwired: 1 in]
              n400 = case shown="\"Square\"" w505 {
                frame "j", Default {
                }
                frame "Sine" {
                  n401 = local write "FGen Waveform"(0) -> ()
                  n402 = local write "Update"(5) -> ()
                  n403 = local write "FGen Waveform"("Sine" ("FGen sWaveform")) -> ()
                }
                frame "Square" {
                  n404 = local write "FGen Waveform"(1) -> ()
                  n405 = local write "Update"(5) -> ()
                  n406 = local write "FGen Waveform"("Square" ("FGen sWaveform")) -> ()
                }
                frame "Triangle" {
                  n407 = local write "FGen Waveform"(2) -> ()
                  n408 = local write "Update"(5) -> ()
                  n409 = local write "FGen Waveform"("Triangle" ("FGen sWaveform")) -> ()
                }
              }
              n410 = Bundle(w514, "JSON Type"=JSON_Type."String") -> (w515:T34)  [unwired: 1 in]
              n411 = Build Array(w515) -> (w512:T35)
              n412 = call <vilib>:"Update Thing Shadow.vi"("Reported State"=w512, "Desired State"=w510, "Thing Shadow in"=w511) -> ()  [unwired: 7 in, 2 out]
            }
            frame "msoSignal" {
              n413 = Pick Line(multi-line string=w529, line index=1) -> (output string=w527:string)  [unwired: 1 in]
              n414 = Pick Line(multi-line string=w529, line index=3) -> (output string=w526:string)  [unwired: 1 in]
              n415 = local write "output string"("") -> ()
              n416 = Bundle("output string"=w527, "output string"=w526) -> (w535:T33)  [unwired: 1 in]
              n417 = case shown="\"Acquire\"" w526 {
                frame "j", Default {
                }
                frame "Acquire" {
                  n418 = local write "Update"(6) -> ()
                  "msoAcquire" <- "Acquire" ("msoAcquire")
                }
              }
              n419 = Bundle(w535, "JSON Type"=JSON_Type."String") -> (w536:T34)  [unwired: 1 in]
              n420 = Build Array(w536) -> (w533:T35)
              n421 = call <vilib>:"Update Thing Shadow.vi"("Reported State"=w533, "Desired State"=w531, "Thing Shadow in"=w532) -> ()  [unwired: 7 in, 2 out]
            }
            frame "reset" {
              n422 = Pick Line(multi-line string=w543, line index=1) -> (output string=w541:string)  [unwired: 1 in]
              n423 = Pick Line(multi-line string=w543, line index=3) -> (output string=w540:string)  [unwired: 1 in]
              n424 = local write "output string"("") -> ()
              n425 = Bundle("output string"=w541, "output string"=w540) -> (w549:T33)  [unwired: 1 in]
              n426 = case shown="\"dio\"" w540 {
                frame "j", Default {
                }
                frame "dio" {
                  n427 = local write "Update"(7) -> ()
                  "Reset" <- "dio" ("msoAcquire")
                }
                frame "mso" {
                  n428 = local write "Update"(7) -> ()
                  n429 = local write "Reset"("mso" ("msoAcquire")) -> ()
                }
              }
              n430 = Bundle(w549, "JSON Type"=JSON_Type."String") -> (w550:T34)  [unwired: 1 in]
              n431 = Build Array(w550) -> (w547:T35)
              n432 = call <vilib>:"Update Thing Shadow.vi"("Reported State"=w547, "Desired State"=w545, "Thing Shadow in"=w546) -> ()  [unwired: 7 in, 2 out]
            }
            frame "usbSignal" {
              n433 = Pick Line(multi-line string=w559, line index=1) -> (output string=w557:string)  [unwired: 1 in]
              n434 = Pick Line(multi-line string=w559, line index=3) -> (output string=w556:string)  [unwired: 1 in]
              n435 = local write "output string"("") -> ()
              n436 = Bundle("output string"=w557, "output string"=w556) -> (w565:T33)  [unwired: 1 in]
              n437 = case shown="\"Acquire\"" w556 {
                frame "j", Default {
                }
                frame "Acquire" {
                  n438 = local write "Update"(8) -> ()
                  "usbAcquire" <- "Acquire" ("msoAcquire")
                }
              }
              n439 = Bundle(w565, "JSON Type"=JSON_Type."String") -> (w566:T34)  [unwired: 1 in]
              n440 = Build Array(w566) -> (w563:T35)
              n441 = call <vilib>:"Update Thing Shadow.vi"("Reported State"=w563, "Desired State"=w561, "Thing Shadow in"=w562) -> ()  [unwired: 7 in, 2 out]
            }
          }
        }
      }
    }
    n442 = case shown="True" "stop" {
      tunnel: w22 -> [_ w39]
      frame False {
      }
      frame True {
        n443 = Bundle("stopProgramme", "True") -> (w42:cluster{string, string})  [unwired: 1 in]
        n444 = Bundle(w42, "JSON Type"=JSON_Type."String") -> (w41:cluster{cluster{string, string}, "JSON Type":T3})  [unwired: 1 in]
        n445 = Build Array(w41) -> (w38:T10)
        n446 = call <vilib>:"Update Thing Shadow.vi"("Reported State"=w38, "Desired State"=w38, "Thing Shadow in"=w39) -> ()  [unwired: 7 in, 2 out]
      }
    }
    n447 = local read "Alexa Stop"() -> (w23:bool)
    n448 = Or(x=w23, y="stop") -> (x .or. y?=w24:bool)
    n449 = call <extravilib>:"Write.vi"("element"="stop") -> ("channel"=w20:T36)  [unwired: 1 out]
  }
  n450 = while {
    tunnel: w3 -> [w570]
    stop <- w572 stop-if-true
    n451 = local read "Update"() -> (w574:i32)
    n452 = call <extravilib>:"Read.vi"("channel"=w570) -> ("element"=w571:bool)  [unwired: 1 in, 1 out]
    n453 = case shown="8" w574 {
      frame 0, Default {
        w586 = FALSE ("Reset")
        n454 = local read "Device Name"() -> (w576:tag)
        n455 = Wait (ms)(milliseconds to wait=u32 1000) -> ()  [unwired: 1 out]
        n456 = call <vilib>:"PS Initialize.vi"("Device Name"=w576, "Reset"=w586) -> ("Instrument Handle Out"=w589:refnum<k21>, "Error Out"=w590:errorcluster)  [unwired: 12 in]
        n457 = call <vilib>:"DMM Initialize.vi"("Device Name"=w576, "Reset"=w586) -> ("Instrument Handle Out"=w585:refnum<k21>, "Error Out"=w584:errorcluster)  [unwired: 12 in]
        n458 = flat-sequence {
          tunnel: [w603] -> w582
          tunnel: [w595] -> w575
          tunnel: w582 -> [w675]
          tunnel: w575 -> [w670]
          frame #0 {
            w614 = 14 ("dimension size")
            w621 = TRUE ("replace all? (F)")
            n459 = local read "VB Name"() -> (w601:string)
            n460 = Concatenate Strings(w601, "/dig/" ("string")) -> (w599:string)
            n461 = Concatenate Strings(w599, "0:7") -> (w597:string)
            n462 = call <vilib>:"Dig Initialize.vi"("Lines"=w597, "Reset"=FALSE) -> ("Instrument Handle Out"=w631:refnum<k21>, "Error Out"=w630:errorcluster)  [unwired: 12 in]
            n463 = call <vilib>:"Dig Query Line Configuration.vi"("Instrument Handle In"=w631, "Error In"=w630) -> ("Instrument Handle Out"=w595:refnum<k21>, "Tristate Lines"=w596:tag)  [unwired: 9 in, 3 out]
            n464 = Search and Replace String(replace all?=w621, input string=w596, search string=w599, replace string="\t") -> (result string=w626:string)  [unwired: 4 in, 3 out]
            n465 = call <vilib>:"Trim Whitespace.vi"("string"=w626) -> ("trimmed string"=w623:string)  [unwired: 1 in]
            n466 = Search and Replace String(replace all?=w621, input string=w623, search string=",", replace string="") -> (result string=w622:string)  [unwired: 4 in, 3 out]
            n467 = Spreadsheet String To Array(format string="%s", spreadsheet string=w622, array type (2D Dbl)=string[] []) -> (array=w619:string[])  [unwired: 1 in]
            n468 = Array Size(array=w619) -> (size(s)=w620:i32)
            n469 = for {
              N: w620 -> [_]
              tunnel: w619 -> [w652] mode=indexing
              tunnel: [w645] -> w617 mode=indexing
              n470 = Search and Replace String(input string=w652, search string=":", replace string="\r") -> (result string=w646:string, number of replacements=w649:i32)  [unwired: 5 in, 2 out]
              n471 = Equal?(x=1, y=w649) -> (x = y?=w647:bool)
              n472 = case shown="False" w647 {
                tunnel: w646 -> [w655 w661]
                tunnel: [w653 w656] -> w645
                frame False {
                  n473 = Decimal String To Number(string=w655) -> (number=w654:i32)  [unwired: 2 in, 1 out]
                  n474 = Build Array(w654) -> (w653:i32[])
                }
                frame True {
                  n475 = Pick Line(multi-line string=w661, line index=1) -> (output string=w659:string)  [unwired: 1 in]
                  n476 = Pick Line(multi-line string=w661, line index=0) -> (output string=w660:string)  [unwired: 1 in]
                  n477 = Decimal String To Number(string=w659) -> (number=w658:i32)  [unwired: 2 in, 1 out]
                  n478 = Decimal String To Number(string=w660) -> (number=w657:i32)  [unwired: 2 in, 1 out]
                  n479 = while {
                    tunnel: w658 -> [w669]
                    tunnel: w657 -> [w666]
                    tunnel: [w664] -> w656 mode=indexing
                    i -> [w667]
                    stop <- w668 continue-if-true
                    n480 = Add(x=w666, y=w667) -> (x+y=w665:i32)
                    n481 = In Range and Coerce(upper limit=w669, x=w665, lower limit=w666) -> (coerced(x)=w664:i32, In Range?=w668:bool)
                  }
                }
              }
            }
            n482 = Reshape Array(w617, w614) -> (w615:i32[])
            n483 = Array Max & Min(array=w617) -> (max value=w616:i32)  [unwired: 3 out]
            n484 = Search 1D Array(1D array=w615, element=w616, start index (0)=1) -> (index of element=w612:i32)
            n485 = Increment(x=w612) -> (x+1=w611:i32)
            n486 = Subtract(x=w614, y=w611) -> (x-y=w613:i32)
            n487 = Delete From Array(array=w615, length=w613, index=w611) -> (array with subset deleted=w610:i32[])  [unwired: 1 out]
            n488 = Number To Decimal String(number=w610) -> (decimal integer string=w609:string[])  [unwired: 1 in]
            n489 = Concatenate Strings(w609) -> (w608:string)
            n490 = Search and Replace String(replace all?=TRUE ("replace all? (F)"), input string=w608, search string="0", replace string="", offset=1 ("offset (0)")) -> (result string=w603:string)  [unwired: 3 in, 3 out]
            n491 = String Length(string=w603) -> (length=w602:i32)
            n492 = for {
              N: w602 -> [_]
              tunnel: w603 -> [w636]
              i -> [w635]
              n493 = String Subset(string=w636, offset (0)=w635, length (rest)=1 ("length (rest)")) -> (substring=w633:string)
              n494 = case shown="\"0\", Default" w633 {
                frame "0", Default {
                  "pin 0" <- "Input"
                }
                frame "1" {
                  "pin 1" <- "Input"
                }
                frame "2" {
                  "pin 2" <- "Input"
                }
                frame "3" {
                  "pin 3" <- "Input"
                }
                frame "4" {
                  "pin 4" <- "Input"
                }
                frame "5" {
                  "pin 5" <- "Input"
                }
                frame "6" {
                  "pin 6" <- "Input"
                }
                frame "7" {
                  "pin 7" <- "Input"
                }
              }
            }
          }
          frame #1 {
            n495 = for {
              N: 8 -> [_]
              tunnel: w675 -> [w759]
              tunnel: [w754] -> w674 mode=indexing
              i -> [w755]
              n496 = String Subset(string="01234567", offset (0)=w755, length (rest)=1 ("length (rest)")) -> (substring=w758:string)
              n497 = Match Pattern(string=w759, regular expression=w758) -> (offset past match=w757:i32)  [unwired: 1 in, 3 out]
              n498 = Greater Or Equal To 0?(x=w757) -> (x >= 0?=w756:bool)
              n499 = case shown="True" w756 {
                tunnel: w755 -> [w764 _]
                tunnel: [w762 ""] -> w754
                frame False {
                  n500 = Number To Decimal String(number=w764, width (-)=i16 1) -> (decimal integer string=w762:string)
                }
                frame True {
                }
              }
            }
            n501 = Concatenate Strings(w674) -> (w672:string)
            n502 = String Length(string=w672) -> (length=w673:i32)
            n503 = for {
              N: w673 -> [_]
              tunnel: w672 -> [w679]
              tunnel: [w677] -> w671
              i -> [w680]
              n504 = String Subset(string=w679, offset (0)=w680, length (rest)=1 ("length (rest)")) -> (substring=w678:string)
              n505 = case shown="\"7\"" w678 {
                tunnel: [w682 w691 w700 w709 w718 w727 w736 w745] -> w677
                frame "0", Default {
                  n506 = local read "VB Name"() -> (w685:string)
                  n507 = Concatenate Strings(w685, "/dig/0" ("string")) -> (w683:string)
                  n508 = call <vilib>:"Dig Read.vi"("Lines"=w683) -> ("Data"=w688:bool[], "Error Out"=w682:errorcluster)  [unwired: 13 in]
                  n509 = Index Array(array=w688, index=0) -> (element=w686:bool)
                  n510 = case shown="True" w686 {
                    frame False {
                      n511 = local write "pin 0"("Low") -> ()
                    }
                    frame True {
                      n512 = local write "pin 0"("High") -> ()
                    }
                  }
                }
                frame "1" {
                  n513 = local read "VB Name"() -> (w694:string)
                  n514 = Concatenate Strings(w694, "/dig/1" ("string")) -> (w692:string)
                  n515 = call <vilib>:"Dig Read.vi"("Lines"=w692) -> ("Data"=w697:bool[], "Error Out"=w691:errorcluster)  [unwired: 13 in]
                  n516 = Index Array(array=w697, index=0) -> (element=w695:bool)
                  n517 = case shown="True" w695 {
                    frame False {
                      n518 = local write "pin 1"("Low") -> ()
                    }
                    frame True {
                      n519 = local write "pin 1"("High") -> ()
                    }
                  }
                }
                frame "2" {
                  n520 = local read "VB Name"() -> (w703:string)
                  n521 = Concatenate Strings(w703, "/dig/2" ("string")) -> (w701:string)
                  n522 = call <vilib>:"Dig Read.vi"("Lines"=w701) -> ("Data"=w706:bool[], "Error Out"=w700:errorcluster)  [unwired: 13 in]
                  n523 = Index Array(array=w706, index=0) -> (element=w704:bool)
                  n524 = case shown="True" w704 {
                    frame False {
                      n525 = local write "pin 2"("Low") -> ()
                    }
                    frame True {
                      n526 = local write "pin 2"("High") -> ()
                    }
                  }
                }
                frame "3" {
                  n527 = local read "VB Name"() -> (w712:string)
                  n528 = Concatenate Strings(w712, "/dig/3" ("string")) -> (w710:string)
                  n529 = call <vilib>:"Dig Read.vi"("Lines"=w710) -> ("Data"=w715:bool[], "Error Out"=w709:errorcluster)  [unwired: 13 in]
                  n530 = Index Array(array=w715, index=0) -> (element=w713:bool)
                  n531 = case shown="True" w713 {
                    frame False {
                      n532 = local write "pin 3"("Low") -> ()
                    }
                    frame True {
                      n533 = local write "pin 3"("High") -> ()
                    }
                  }
                }
                frame "4" {
                  n534 = local read "VB Name"() -> (w721:string)
                  n535 = Concatenate Strings(w721, "/dig/4" ("string")) -> (w719:string)
                  n536 = call <vilib>:"Dig Read.vi"("Lines"=w719) -> ("Data"=w724:bool[], "Error Out"=w718:errorcluster)  [unwired: 13 in]
                  n537 = Index Array(array=w724, index=0) -> (element=w722:bool)
                  n538 = case shown="True" w722 {
                    frame False {
                      n539 = local write "pin 4"("Low") -> ()
                    }
                    frame True {
                      n540 = local write "pin 4"("High") -> ()
                    }
                  }
                }
                frame "5" {
                  n541 = local read "VB Name"() -> (w730:string)
                  n542 = Concatenate Strings(w730, "/dig/5" ("string")) -> (w728:string)
                  n543 = call <vilib>:"Dig Read.vi"("Lines"=w728) -> ("Data"=w733:bool[], "Error Out"=w727:errorcluster)  [unwired: 13 in]
                  n544 = Index Array(array=w733, index=0) -> (element=w731:bool)
                  n545 = case shown="False" w731 {
                    frame False {
                      n546 = local write "pin 5"("Low") -> ()
                    }
                    frame True {
                      n547 = local write "pin 5"("High") -> ()
                    }
                  }
                }
                frame "6" {
                  n548 = local read "VB Name"() -> (w739:string)
                  n549 = Concatenate Strings(w739, "/dig/6" ("string")) -> (w737:string)
                  n550 = call <vilib>:"Dig Read.vi"("Lines"=w737) -> ("Data"=w742:bool[], "Error Out"=w736:errorcluster)  [unwired: 13 in]
                  n551 = Index Array(array=w742, index=0) -> (element=w740:bool)
                  n552 = case shown="True" w740 {
                    frame False {
                      n553 = local write "pin 6"("Low") -> ()
                    }
                    frame True {
                      n554 = local write "pin 6"("High") -> ()
                    }
                  }
                }
                frame "7" {
                  n555 = local read "VB Name"() -> (w748:string)
                  n556 = Concatenate Strings(w748, "/dig/7" ("string")) -> (w746:string)
                  n557 = call <vilib>:"Dig Read.vi"("Lines"=w746) -> ("Data"=w751:bool[], "Error Out"=w745:errorcluster)  [unwired: 13 in]
                  n558 = Index Array(array=w751, index=0) -> (element=w749:bool)
                  n559 = case shown="False" w749 {
                    frame False {
                      n560 = local write "pin 7"("Low") -> ()
                    }
                    frame True {
                      n561 = local write "pin 7"("High") -> ()
                    }
                  }
                }
              }
            }
            n562 = call <vilib>:"Dig Close.vi"("Instrument Handle In"=w670, "Error In"=w671) -> ()  [unwired: 13 in, 1 out]
          }
        }
        n563 = call <vilib>:"DMM Query Measurement.vi"("Instrument Handle In"=w585, "Error In"=w584) -> ("Instrument Handle Out"=w578:refnum<k21>, "Function"=w583:i32, "Auto Range"=w588:bool, "Range"=→"DMM Range":dbl, "Error Out"=w579:errorcluster)  [unwired: 9 in]
        n564 = for {
          N: 3 -> [_]
          tunnel: w589 -> [w786]
          tunnel: w590 -> [w785]
          tunnel: [w784] -> w592
          tunnel: [w783] -> w591
          i -> [w782]
          w775 = 0.001
          n565 = case shown="0, Default" w782 {
            tunnel: [tag "ps/+6V" ("Channel") tag "ps/+25V" ("Channel") tag "ps/-25V" ("Channel")] -> w787
            frame 0, Default {
            }
            frame 1 {
            }
            frame 2 {
            }
          }
          n566 = call <vilib>:"PS Query Voltage Output.vi"("Instrument Handle In"=w786, "Channel"=w787, "Error In"=w785) -> ("Instrument Handle Out"=w783:refnum<k21>, "Voltage Level"=w780:dbl, "Current Limit"=w774:dbl, "Error Out"=w784:errorcluster)  [unwired: 9 in]
          n567 = Divide(x=w780, y=w775) -> (x/y=w776:dbl)
          n568 = Divide(x=w774, y=w775) -> (x/y=w777:dbl)
          n569 = Round To Nearest(number=w776) -> (nearest integer value=w781:dbl)
          n570 = Round To Nearest(number=w777) -> (nearest integer value=w778:dbl)
          n571 = Multiply(x=w781, y=w775) -> (x*y=w779:dbl)
          n572 = Multiply(x=w778, y=w775) -> (x*y=w773:dbl)
          n573 = case shown="0, Default" w782 {
            tunnel: w779 -> [w789 w791 w793]
            tunnel: w773 -> [w788 w790 w792]
            frame 0, Default {
              n574 = local write "Voltage C1"(w789) -> ()
              n575 = local write "Current C1"(w788) -> ()
            }
            frame 1 {
              n576 = local write "Voltage C2"(w791) -> ()
              n577 = local write "Current C2"(w790) -> ()
            }
            frame 2 {
              n578 = local write "Voltage C3"(w793) -> ()
              n579 = local write "Current C3"(w792) -> ()
            }
          }
        }
        n580 = case shown="0, Default" w583 {
          frame 0, Default {
            n581 = local write "DMM Function String"("DC Volts") -> ()
          }
          frame 1 {
            n582 = local write "DMM Function String"("AC Volts") -> ()
          }
          frame 2 {
            n583 = local write "DMM Function String"("DC Current") -> ()
          }
          frame 3 {
            n584 = local write "DMM Function String"("AC Current") -> ()
          }
          frame 4 {
            n585 = local write "DMM Function String"("Resistance") -> ()
          }
          frame 5 {
            n586 = local write "DMM Function String"("Diode") -> ()
          }
          frame 6 {
            n587 = local write "DMM Function String"("Continuity") -> ()
          }
        }
        n588 = local write "Auto Range"(w588) -> ()
        n589 = local write "DMM Function"(w583) -> ()
        n590 = call <vilib>:"DMM Read.vi"("Instrument Handle In"=w578, "Error In"=w579) -> ("Instrument Handle Out"=w580:refnum<k21>, "Measurement"=→"DMM Measurement":dbl, "Error Out"=w581:errorcluster)  [unwired: 11 in]
        n591 = call <vilib>:"DMM Close.vi"("Instrument Handle In"=w580, "Error In"=w581) -> ()  [unwired: 13 in, 1 out]
        n592 = call <vilib>:"PS Close.vi"("Instrument Handle In"=w591, "Error In"=w592) -> ()  [unwired: 13 in, 1 out]
      }
      frame 1 {
        n593 = local write "Update"(0) -> ()
        n594 = local read "Device Name"() -> (w800:tag)
        n595 = local read "Voltage Update Value"() -> (w803:dbl)
        n596 = local read "Voltage Channel"() -> (w804:tag)
        n597 = call <vilib>:"PS Initialize.vi"("Device Name"=w800, "Reset"=FALSE) -> ("Instrument Handle Out"=w798:refnum<k21>, "Error Out"=w797:errorcluster)  [unwired: 12 in]
        n598 = call-poly <vilib>:"PS Configure Voltage Output.vi"("Instrument Handle In"=w798, "Channel"=w804, "Voltage Level"=w803, "Error In"=w797) -> ("Instrument Handle Out"=w805:refnum<k21>, "Error Out"=w802:errorcluster)  [unwired: 10 in]
        n599 = call <vilib>:"PS Close.vi"("Instrument Handle In"=w805, "Error In"=w802) -> ()  [unwired: 13 in, 1 out]
      }
      frame 2 {
        n600 = local write "Update"(0) -> ()
        n601 = local read "Device Name"() -> (w809:tag)
        n602 = local read "Current Update Value"() -> (w810:dbl)
        n603 = local read "Voltage Channel"() -> (w813:tag)
        n604 = call <vilib>:"PS Initialize.vi"("Device Name"=w809, "Reset"=FALSE) -> ("Instrument Handle Out"=w807:refnum<k21>, "Error Out"=w806:errorcluster)  [unwired: 12 in]
        n605 = call-poly <vilib>:"PS Configure Voltage Output.vi"("Instrument Handle In"=w807, "Channel"=w813, "Current Limit"=w810, "Error In"=w806) -> ("Instrument Handle Out"=w814:refnum<k21>, "Error Out"=w811:errorcluster)  [unwired: 10 in]
        n606 = call <vilib>:"PS Close.vi"("Instrument Handle In"=w814, "Error In"=w811) -> ()  [unwired: 13 in, 1 out]
      }
      frame 3 {
        n607 = local write "Update"(0) -> ()
        n608 = local read "Device Name"() -> (w817:tag)
        n609 = local read "DMM Function"() -> (w822:i32)
        n610 = call <vilib>:"DMM Initialize.vi"("Device Name"=w817, "Reset"=FALSE) -> ("Instrument Handle Out"=w816:refnum<k21>, "Error Out"=w815:errorcluster)  [unwired: 12 in]
        n611 = call-poly <vilib>:"DMM Configure Measurement.vi"("Instrument Handle In"=w816, "Function"=w822, "Error In"=w815) -> ("Instrument Handle Out"=w821:refnum<k21>, "Error Out"=w820:errorcluster)  [unwired: 11 in]
        n612 = call <vilib>:"DMM Close.vi"("Instrument Handle In"=w821, "Error In"=w820) -> ()  [unwired: 13 in, 1 out]
      }
      frame 4 {
        n613 = local read "DIOPins"() -> (w827:tag)
        n614 = local read "DIOUpdateValue"() -> (w829:string)
        n615 = local write "Update"(0) -> ()
        n616 = call <vilib>:"Dig Initialize.vi"("Lines"=w827, "Reset"=FALSE) -> ("Instrument Handle Out"=w824:refnum<k21>, "Error Out"=w826:errorcluster)  [unwired: 12 in]
        n617 = case shown="\"Input\"" w829 {
          tunnel: w827 -> [w835 w843 w849]
          tunnel: w826 -> [w834 w841 w850]
          tunnel: [w833 w840 w846] -> w825
          tunnel: w824 -> [w836 w842 w848]
          tunnel: [w832 w839 w847] -> w823
          frame "High", Default {
            n618 = Wait (ms)(milliseconds to wait=u32 50) -> ()  [unwired: 1 out]
            n619 = call <vilib>:"Dig Write.vi"("Instrument Handle In"=w836, "Lines"=w835, "Data"=bool[] [TRUE], "Error In"=w834) -> ("Instrument Handle Out"=w832:refnum<k21>, "Error Out"=w833:errorcluster)  [unwired: 10 in]
          }
          frame "Low" {
            n620 = Wait (ms)(milliseconds to wait=u32 50) -> ()  [unwired: 1 out]
            n621 = call <vilib>:"Dig Write.vi"("Instrument Handle In"=w842, "Lines"=w843, "Data"=bool[] [FALSE], "Error In"=w841) -> ("Instrument Handle Out"=w839:refnum<k21>, "Error Out"=w840:errorcluster)  [unwired: 10 in]
          }
          frame "Input" {
            n622 = call <vilib>:"Dig Tristate Lines.vi"("Instrument Handle In"=w848, "Lines"=w849, "Error In"=w850) -> ("Instrument Handle Out"=w847:refnum<k21>, "Error Out"=w846:errorcluster)  [unwired: 11 in]
            n623 = Wait (ms)(milliseconds to wait=u32 50) -> ()  [unwired: 1 out]
          }
        }
        n624 = call <vilib>:"Dig Close.vi"("Instrument Handle In"=w823, "Error In"=w825) -> ()  [unwired: 13 in, 1 out]
      }
      frame 5 {
        n625 = local read "Device Name"() -> (w851:tag)
        n626 = local read "FGen Waveform"() -> (w852:i32)
        n627 = local write "Update"(0) -> ()
        n628 = call <vilib>:"FGEN Initialize.vi"("Device Name"=w851) -> ("Instrument Handle Out"=w858:refnum<k21>, "Error Out"=w857:errorcluster)  [unwired: 13 in]
        n629 = call-poly <vilib>:"FGEN Configure Standard Waveform.vi"("Instrument Handle In"=w858, "Waveform Function"=w852, "Error In"=w857) -> ("Instrument Handle Out"=w855:refnum<k21>, "Error Out"=w856:errorcluster)  [unwired: 11 in]
        n630 = call <vilib>:"FGEN Run.vi"("Instrument Handle In"=w855, "Error In"=w856) -> ("Instrument Handle Out"=w854:refnum<k21>, "Error Out"=w853:errorcluster)  [unwired: 12 in]
        n631 = call <vilib>:"FGEN Close.vi"("Instrument Handle In"=w854, "Error In"=w853) -> ()  [unwired: 13 in, 1 out]
      }
      frame 6 {
        w861 = TRUE ("replace all? (F)")
        n632 = local write "Update"(0) -> ()
        n633 = Get Date/Time String(want seconds? (F)=TRUE) -> (date string=w872:string, time string=w865:string)  [unwired: 2 in]
        n634 = local read "Device Name"() -> (w884:tag)
        n635 = Search and Replace String(replace all?=w861, input string=w865, search string=":") -> (result string=w863:string)  [unwired: 5 in, 3 out]
        n636 = Search and Replace String(replace all?=w861, input string=w872, search string="/") -> (result string=w870:string)  [unwired: 5 in, 3 out]
        n637 = call <vilib>:"MSO Initialize.vi"("Device Name"=w884, "Reset"=FALSE) -> ("Instrument Handle Out"=w878:refnum<k21>, "Error Out"=w877:errorcluster)  [unwired: 12 in]
        n638 = Concatenate Strings("C:\\Users\\Joe\\Documents\\Final Year Project\\Waveforms\\VBWaveform_", w870, "_", w863, ".xls") -> (w867:string)
        n639 = call <vilib>:"MSO Run.vi"("Instrument Handle In"=w878, "Auto Trigger"=TRUE, "Error In"=w877) -> ("Instrument Handle Out"=w882:refnum<k21>, "Error Out"=w883:errorcluster)  [unwired: 11 in]
        n640 = local write "msoAcquire"("Ready") -> ()
        n641 = String To Path(string=w867) -> (path=w866:path)
        n642 = call <vilib>:"MSO Read.vi"("Instrument Handle In"=w882, "Error In"=w883) -> ("Instrument Handle Out"=w881:refnum<k21>, "Analog Waveforms"=w875:waveform(dbl)[], "Error Out"=w880:errorcluster)  [unwired: 8 in, 3 out]
        n643 = call <vilib>:"MSO Close.vi"("Instrument Handle In"=w881, "Error In"=w880) -> ()  [unwired: 13 in, 1 out]
        n644 = call-poly <vilib>:"Export Waveforms to Spreadsheet File.vi"("waveforms"=w875, "file path (dialog if empty)"=w866) -> ("error out"=w874:errorcluster)  [unwired: 8 in, 1 out]
        n645 = call <vilib>:"Simple Error Handler.vi"("error in (no error)"=w874) -> ()  [unwired: 4 in, 5 out]
      }
      frame 7 {
        n646 = local read "Reset"() -> (w886:string)
        n647 = local write "Update"(0) -> ()
        n648 = case shown="\"dio\"" w886 {
          frame "mso" {
            n649 = local read "Device Name"() -> (w890:tag)
            n650 = call <vilib>:"MSO Initialize.vi"("Device Name"=w890, "Reset"=FALSE) -> ("Instrument Handle Out"=w894:refnum<k21>, "Error Out"=w893:errorcluster)  [unwired: 12 in]
            n651 = local write "Reset"("Ready") -> ()
            n652 = call <vilib>:"MSO Reset Instrument.vi"("Instrument Handle In"=w894, "Error In"=w893) -> ("Instrument Handle Out"=w891:refnum<k21>, "Error Out"=w892:errorcluster)  [unwired: 12 in]
            n653 = call <vilib>:"MSO Close.vi"("Instrument Handle In"=w891, "Error In"=w892) -> ()  [unwired: 13 in, 1 out]
          }
          frame "dio" {
            n654 = flat-sequence {
              tunnel: [w905] -> w896
              tunnel: [w904] -> w895
              tunnel: w896 -> [w909]
              tunnel: w895 -> [w908]
              frame #0 {
                w906 = "Input"
                n655 = local read "VB Name"() -> (w902:string)
                n656 = Concatenate Strings(w902, "/dig/0:7" ("string")) -> (w898:string)
                n657 = call <vilib>:"Dig Initialize.vi"("Lines"=w898, "Reset"=FALSE) -> ("Instrument Handle Out"=w899:refnum<k21>, "Error Out"=w897:errorcluster)  [unwired: 12 in]
                n658 = call <vilib>:"Dig Tristate Lines.vi"("Instrument Handle In"=w899, "Lines"=w898, "Error In"=w897) -> ("Instrument Handle Out"=w904:refnum<k21>, "Error Out"=w905:errorcluster)  [unwired: 11 in]
                n659 = local write "pin 6"(w906) -> ()
                n660 = local write "pin 0"(w906) -> ()
                n661 = local write "pin 1"(w906) -> ()
                n662 = local write "pin 2"(w906) -> ()
                n663 = local write "pin 3"(w906) -> ()
                n664 = local write "pin 4"(w906) -> ()
                n665 = local write "pin 5"(w906) -> ()
                n666 = local write "pin 7"(w906) -> ()
                n667 = Wait (ms)(milliseconds to wait=u32 100) -> ()  [unwired: 1 out]
              }
              frame #1 {
                n668 = call <vilib>:"Dig Close.vi"("Instrument Handle In"=w908, "Error In"=w909) -> ()  [unwired: 13 in, 1 out]
                n669 = local write "Reset"("Ready") -> ()
              }
            }
          }
          frame "j", Default {
          }
        }
      }
      frame 8 {
        w912 = TRUE ("replace all? (F)")
        w926 = 100
        w929 = -1 items=["Default"=-1, "RSE"=10083, "NRSE"=10078, "Differential"=10106, "Pseudodifferential"=12529] ("input terminal configuration")
        w937 = 10123 items=["Finite Samples"=10178, "Continuous Samples"=10123, "Hardware Timed Single Point"=12522]  # Sample Mode
        w938 = T37 3 items=["no dialog", "OK message", "continue or stop message", "OK message + warnings", "continue/stop + warnings"] ("type of dialog (OK msg:1)")
        n670 = local write "Update"(0 ("Update")) -> ()
        n671 = call-poly <vilib>:"DAQmx Create Virtual Channel.vi"("maximum value"=5.0, "minimum value"=-5.0, "input terminal configuration"=w929, "physical channels"="Physical Channel") -> ("task out"=w935:refnum<k21>, "error out"=w936:errorcluster)  [unwired: 10 in]
        n672 = call-poly <vilib>:"DAQmx Timing.vi"("task/channels in"=w935, "sample mode"=w937, "samples per channel"=w926, "rate"=1000.0, "source"=tag "OnboardClock", "error in"=w936) -> ("task out"=w933:refnum<k21>, "error out"=w932:errorcluster)  [unwired: 8 in]
        n673 = call <vilib>:"DAQmx Start Task.vi"("task/channels in"=w933, "error in"=w932) -> ("task out"=w945:refnum<k21>, "error out"=w944:errorcluster)  [unwired: 12 in]
        n674 = local write "usbAcquire"("Ready") -> ()
        n675 = while {
          tunnel: w945 -> [w957]
          tunnel: w944 -> [w956]
          tunnel: [w953] -> w941
          tunnel: [w954] -> w942
          tunnel: w926 -> [w951]
          tunnel: [w950] -> w911
          stop <- w955 stop-if-true
          n676 = call-poly <vilib>:"DAQmx Read.vi"("task/channels in"=w957, "number of samples per channel"=w951, "error in"=w956) -> ("task out"=w954:refnum<k21>, "data"=w950:waveform(dbl)[], "error out"=w953:errorcluster)  [unwired: 10 in]
          n677 = Tick Count (ms)() -> (millisecond timer value=w948:u32)
          n678 = Greater Or Equal?(x=w948, y=100) -> (x >= y?=w947:bool)
          n679 = Unbundle By Name(w953) -> ("status"=w952:bool)
          n680 = Or(x=w952, y=w947) -> (x .or. y?=w955:bool)
        }
        n681 = call <vilib>:"DAQmx Stop Task.vi"("task/channels in"=w942, "error in"=w941) -> ("task out"=w940:refnum<k21>, "error out"=w939:errorcluster)  [unwired: 12 in]
        n682 = call <vilib>:"DAQmx Clear Task.vi"("task in"=w940, "error in"=w939) -> ("error out"=w943:errorcluster)  [unwired: 13 in]
        n683 = Get Date/Time String(want seconds? (F)=TRUE) -> (date string=w923:string, time string=w916:string)  [unwired: 2 in]
        n684 = call <vilib>:"Simple Error Handler.vi"("type of dialog (OK msg:1)"=w938, "error in (no error)"=w943) -> ()  [unwired: 3 in, 5 out]
        n685 = Search and Replace String(replace all?=w912, input string=w916, search string=":") -> (result string=w914:string)  [unwired: 5 in, 3 out]
        n686 = Search and Replace String(replace all?=w912, input string=w923, search string="/") -> (result string=w921:string)  [unwired: 5 in, 3 out]
        n687 = Concatenate Strings("C:\\Users\\Joe\\Documents\\Final Year Project\\Waveforms\\USBWaveform_", w921, "_", w914, ".xls") -> (w918:string)
        n688 = String To Path(string=w918) -> (path=w917:path)
        n689 = call-poly <vilib>:"Export Waveforms to Spreadsheet File.vi"("waveforms"=w911, "file path (dialog if empty)"=w917) -> ("error out"=w924:errorcluster)  [unwired: 8 in, 1 out]
        n690 = call <vilib>:"Simple Error Handler.vi"("error in (no error)"=w924) -> ()  [unwired: 4 in, 5 out]
      }
    }
    n691 = local read "Alexa Stop"() -> (w573:bool)
    n692 = Or(x=w571, y=w573) -> (x .or. y?=w572:bool)
  }
  "Voltage Update Value" <- w7
  "Update" <- w8
  "Current Update Value" <- w7
  "Device Name" <- w2
  "Alexa Stop" <- FALSE
  "stopProgramme" <- "False"
  "FGen Waveform" <- w8
  "VB Name" <- w2
